vi "TLB Native Dynamic Events ver 0.13g.vi"() -> ()   [LabVIEW 2018]
uses:
  Labview Training Phase 2/Enum Controls/States for Action Engine.ctl
  TLB Type Definitions/State Type Definitions.ctl
  TLB Type Definitions/Intruction Type Definitions.ctl
  TLB Type Definitions/Encoder cluster.ctl
  TLB Type Definitions/PING CLUSTER.ctl
  <vilib>/Studica/Studica Toolkit/NavX/NavX.lvlib
  <vilib>/Studica/Studica Toolkit/Background/DIO Channel.ctl
  Underlying VI's/NavX VI/navX type def.ctl
  <vilib>/myRIO/Instrument Drivers/Utilities/Utilities.lvlib
  <vilib>/Studica/Studica Toolkit/Background/I2C Channel.ctl
  TLB Type Definitions/Vision cluster.ctl
  <vilib>/NI_Real-Time Target Support.lvlib
  TLB Type Definitions/Stepper cluster.ctl
  Experimental VI's/Archived VI's/MOTOR CONTROL NO PID Type Def.ctl
  Underlying VI's/I2C Master VI/I2C MASTER Type Def.ctl
  Underlying VI's/I2C Master VI/I2C_MASTER_WRITE_NEW Type Def.ctl
  Underlying VI's/Webcam FGV Low level ver/State control.ctl
  <vilib>/userdefined/High Color/IMAQdx.ctl
  Underlying VI's/I2C Master VI/Arduino_Interfacing.ctl
  TLB Type Definitions/Yaw Cluster.ctl
  Experimental VI's/Archived VI's/MOTOR CONTROL NO PID AE DATA ENTRY MODE Type def.ctl
  Experimental VI's/Archived VI's/MOTOR CONTROL NO PID AE DIRECTIONS type def.ctl
  Underlying VI's/Elasped Timer/Control.ctl
  TLB Type Definitions/Time cluster.ctl
  TLB Type Definitions/Y Stepper cluster.ctl
  <vilib>/Utility/RT CPU Load.ctl
panel:
  out "Time up flag":bool
  out "Recognized object + Time up?":bool
  out "Speed & distance":T1
  out "Task selection":u8
  out "Object Center Coordinates":cluster{"x":sgl, "y":sgl}
  out "Object detection cluster":T2
  in  "Object recognition mode":enum16{"Ball", "Soap", "Gel", "Pipe", "None"}(ring)
  out "NavX Readings":T3
  out "Arduino Data":T4
  out "CPU loads":T5[](array[typedef]) {"ISR (%)" format="%#.2f"; "Idle (%)" format="%#.2f"; "Background (%)" format="%#.2f"; "Normal (%)" format="%#.2f"; "Above Normal (%)" format="%#.2f"; "High (%)" format="%#.2g"; "Timed Structures (%)" format="%#.2g"; "Time Critical (%)" format="%#.2g"; "Total (%)" format="%#.2g"}
  in  "Red LED":bool
  out "Obstacle detected?":bool
  out "TASK ENABLE":bool
  out "Rising Edge":bool
  in  "Green LED":bool
  out "Obstacle detected":bool
  out "I2C Error":errorcluster
  out "State Logic":T6=enum."Startup"
  out "elements":T7[](array[typedef])
  in  "STOP TASK":bool
  in  "OK Button":bool
  in  "STOP":bool
  out "error out":errorcluster
  out "Action Queue Items":i32
  out "State Logic Queue Items":i32
  out "Action Queues items":string[](array[string])=["Hardware reset", "Software reset", ""]
  out "Action State":string
  # "System Health Status Update"
  # "TLB FRAMEWORK STATUS"
  # "Test Programme written by Calvin Loke    Dated: 28 Aug 2019\nTest Programme revised by Dr Alex See   Dated 30 Aug 2019\n\nRevision date: 19/03/2020\nProgramme version:   TLB Native Dynamic Events ver 0.13g"
  # "VISION"
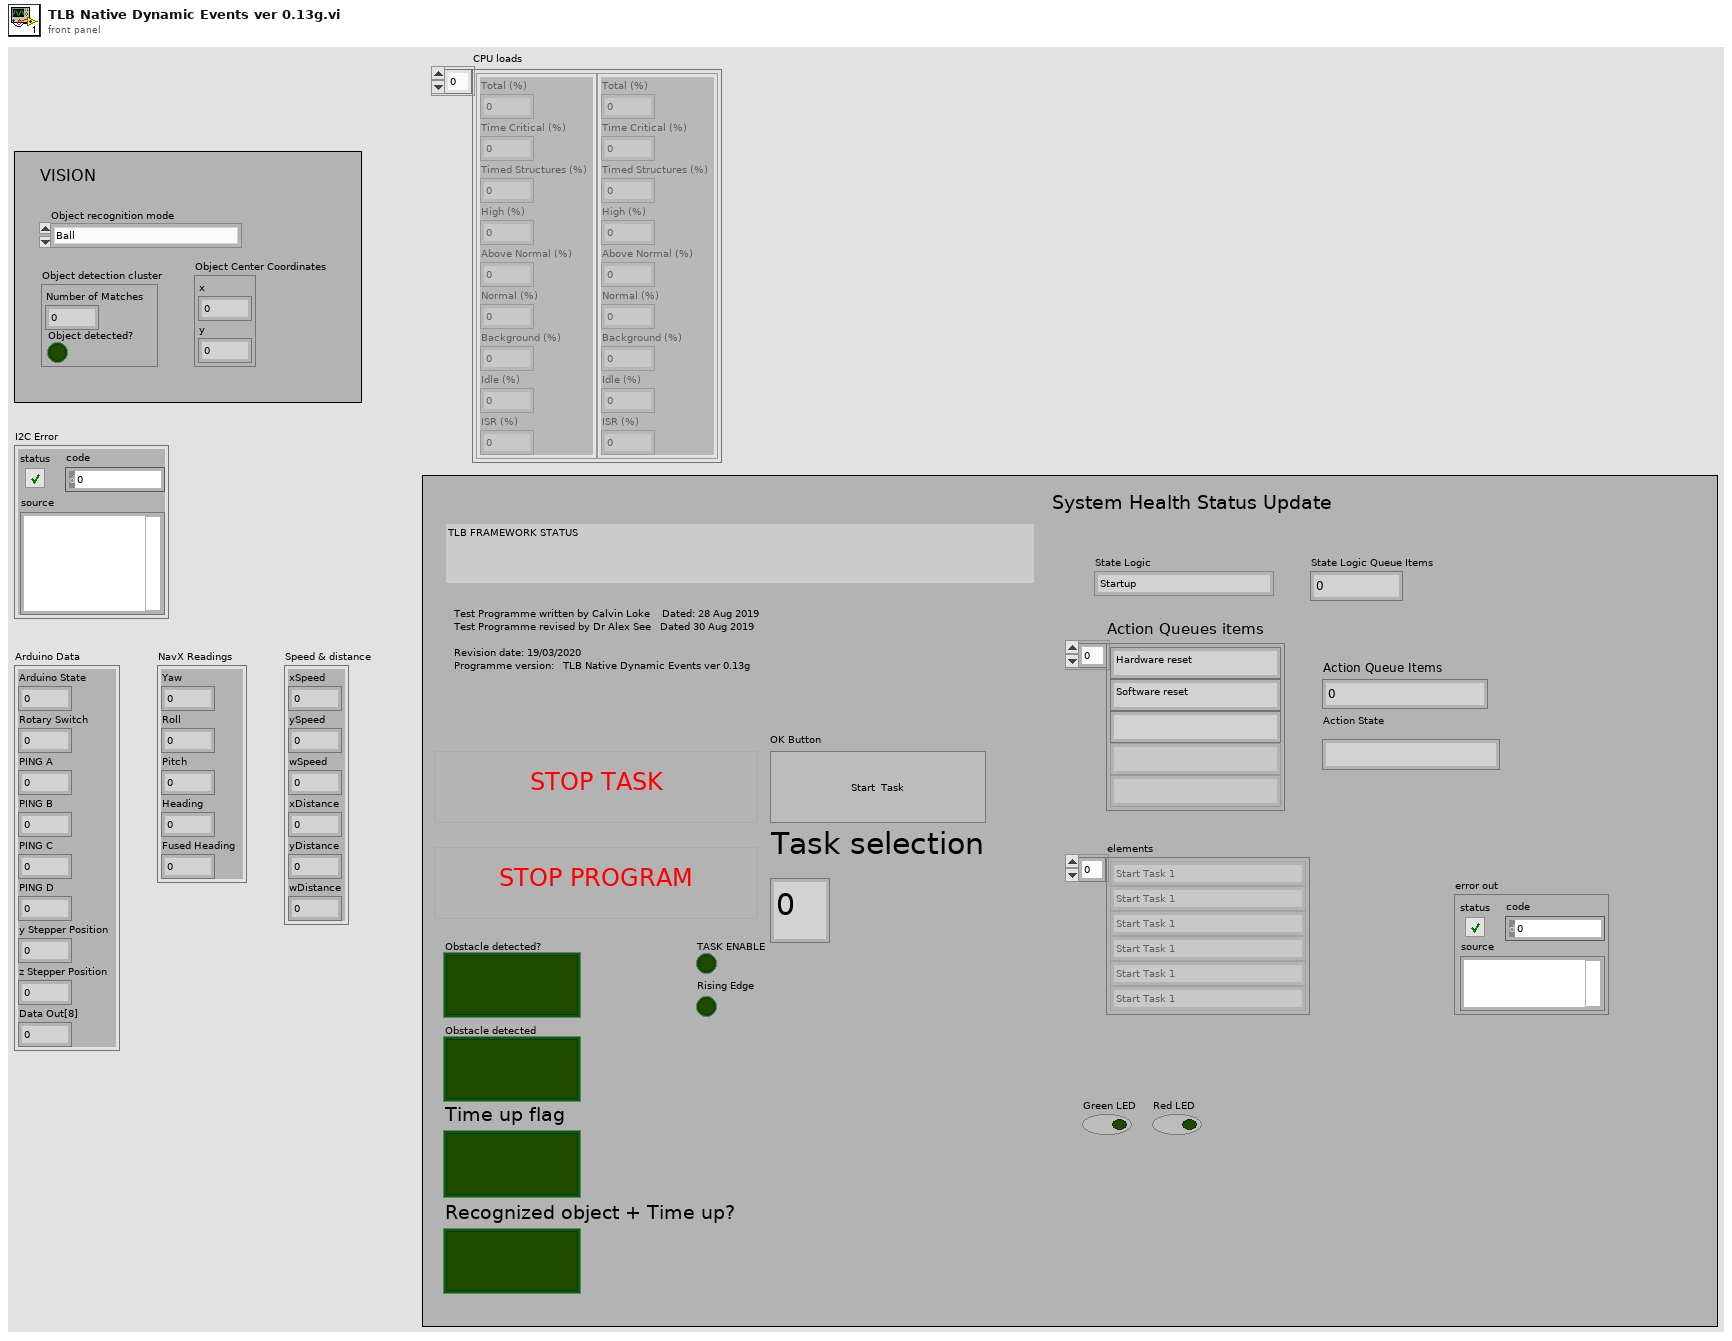
[diagram p1: front panel]
types:
  T1 = cluster{"xSpeed":dbl, "ySpeed":dbl, "wSpeed":dbl, "xDistance":dbl, "yDistance":dbl, "wDistance":dbl}
  T2 = cluster{"Number of Matches":i32, "Object detected?":bool}
  T3 = cluster{"Yaw":dbl, "Roll":dbl, "Pitch":dbl, "Heading":dbl, "Fused Heading":dbl}
  T4 = cluster{"Arduino State":u8, "Rotary Switch":u8, "PING A":u8, "PING B":u8, "PING C":u8, "PING D":u8, "y Stepper Position":u8, "z Stepper Position":u8, "Data Out[8]":u8}
  T5 = typedef "NI_Real-Time Target Support.lvlib/RT CPU Load.ctl" = cluster{"Total (%)":dbl, "Time Critical (%)":dbl, "Timed Structures (%)":dbl, "High (%)":dbl, "Above Normal (%)":dbl, "Normal (%)":dbl, "Background (%)":dbl, "Idle (%)":dbl, "ISR (%)":dbl}
  T6 = typedef "State Type Definitions.ctl" = enum16{"None", "Startup", "Move to Angle", "True Stop", "Idle", "Shutdown", "Task 1A", "Task 1B", "Task 2:Raise Arm", "Task 2:Sensor Mode", "Task 2:Reverse Mode", "Task 3", "Task 4_A", "Task 4_B", "Task 4_C", "Task 4_D", "Task 5A", "Task 5B", "Task 5C", "Task 5D", "Task 5E: POSITION ARM", "Task 5F: ARM GRAB HEIGHT", "Task 5G: CLOSE CLAW", "Task 5H: RAISE ARM", "Task 6_A", "Task 6_B", "Task 7", "Task 8A: RAISE ARM", "Task 8B: MOVE TO BOX", "Task 8C: CAM BURST", "Task 8D: PROCESS IMAGE", "Task 8E: ROBOT ADJUST", "Task 8F: CAM BURST 2", "Task 8G: PROCESS IMAGE 2", "Task 8H: ARM ADJUST", "Task 8I: ARM GRAB HEIGHT", "Task 8J: CLOSE CLAW", "Task 8K: RAISE MY SWORD", "Task 9A: Raise Arm", "Task 9B: Rotate to Angle", "Task 9C: Detect Box", "Task 9D: MOVE FORWARD", "Task 9E: MOVE LEFT", "Task 9F: SCAN IMAGE", "Task 9G: PROCESS COLOUR", "Task 9H: MOVE RIGHT", "Task 9I: SCAN IMAGE", "Task 9J: PROCESS COLOUR", "Task 9K: ROTATE 90 CW", "Task 9L: MOVE FORWARD", "Task 9M: MOVE RIGHT", "Task 9N: SCAN IMAGE", "Task 9O: PROCESS COLOUR", "Task 9P: MOVE RIGHT", "Task 9Q: SCAN IMAGE", "Task 9R: PROCESS COLOUR", "Task A1: Raise Arm", "Task A2: Rotate to Angle", "Task A3: Move Forward", "Task A4: Rotate CW 90"}
  T7 = typedef "Intruction Type Definitions.ctl" = enum16{"None", "Start Task 1", "Start Task 2", "Start Task 3", "Start Task 4", "Start Task 5", "Start Task 6", "Start Task 7", "Start Task 8 - BALL", "Start Task 8 - Gel", "Start Task 8 - Pipe", "Start Task 8 - Soap", "Start Task 9", "Start Task A", "Start Task B", "Exit"}
  T8 = typedef "Y Stepper cluster.ctl" = cluster{"yStepper desired":u8}
  T9 = typedef "Time cluster.ctl" = cluster{"Time up flag":bool, "SET TIME TO CHECK":dbl}
  T10 = typedef "Yaw Cluster.ctl" = cluster{"Yaw":dbl, "Compass":dbl}
  T11 = typedef "Stepper cluster.ctl" = cluster{"y Stepper Position":u8, "z Stepper Position":u8}
  T12 = typedef "DIO Channel.ctl" = enum16{"Not Connected", "A/DIO1", "A/DIO2", "A/DIO3", "A/DIO4", "A/DIO5", "A/DIO6", "A/DIO7", "A/DIO13", "B/DIO1", "B/DIO2", "B/DIO3", "B/DIO4", "B/DIO5", "B/DIO6", "B/DIO7", "B/DIO13", "C/DIO0", "C/DIO1", "C/DIO2", "C/DIO3", "C/DIO4", "C/DIO5", "C/DIO6", "C/DIO7"}
  T13 = typedef "Vision cluster.ctl" = cluster{"Recognized Object":bool, "Object X coordinate":dbl, "Object Y coordinate":dbl}
  T14 = typedef "PING CLUSTER.ctl" = cluster{"PING_A":u8, "PING_B":u8, "PING_C":u8, "PING_D":u8}
  T15 = typedef "Encoder cluster.ctl" = cluster{"xDistance":dbl, "yDistance":dbl, "wDistance":dbl}
  T16 = cluster{"DIO Channel":T12, "FPGA VI Reference Out":refnum<k20>}
  T17 = typedef "MOTOR CONTROL NO PID AE DATA ENTRY MODE Type def.ctl" = enum16{"Initialize", "Reset Encoders", "Write to motors", "Read from Encoders"}
  T18 = typedef "navX type def.ctl" = enum16{"Get i2C reference", "Read Values", "Zero Yaw"}
  T19 = typedef "Arduino_Interfacing.ctl" = enum16{"Initialize", "Write to Arduino", "Read From Arduino"}
  T20 = typedef "I2C Channel.ctl" = enum16{"Not Connected", "A", "B"}
  T21 = typedef "States for Action Engine.ctl" = enum16{"Initialize", "Write", "Read"}
  T22 = cluster{"I2C Ref Out":cluster{"I2C Channel":T20, "FPGA VI Reference Out":refnum<k20>}, "Connected":bool, "Slave Address (7-bit)":u8, "Registry":u8[]}
  T23 = typedef "IMAQ Image.ctl" = refnum<image>
  T24 = typedef "State Type Definitions.ctl" = enum16{"None", "Startup", "Move to Angle", "True Stop", "Idle", "Shutdown", "Task 1", "Task 2:Raise Arm", "Task 2:Sensor Mode", "Task 2:Reverse Mode", "Task 3", "Task 4_A", "Task 4_B", "Task 4_C", "Task 4_D", "Task 5A: ARM CAM HEIGHT", "Task 5B: MOVE TO BOX", "Task 5C: CAM BURST", "Task 5D: PROCESS IMAGE", "Task 5E: POSITION ARM", "Task 5F: ARM GRAB HEIGHT", "Task 5G: CLOSE CLAW", "Task 5H: RAISE ARM", "Task 6_A", "Task 6_B", "Task 7", "Task 8A: RAISE ARM", "Task 8B: MOVE TO BOX", "Task 8C: CAM BURST", "Task 8D: PROCESS IMAGE", "Task 8E: ROBOT ADJUST", "Task 8F: CAM BURST 2", "Task 8G: PROCESS IMAGE 2", "Task 8H: ARM ADJUST", "Task 8I: ARM GRAB HEIGHT", "Task 8J: CLOSE CLAW", "Task 8K: RAISE MY SWORD", "Task 9A: Raise Arm", "Task 9B: Rotate to Angle", "Task 9C: Detect Box", "Task 9D: MOVE FORWARD", "Task 9E: MOVE LEFT", "Task 9F: SCAN IMAGE", "Task 9G: PROCESS COLOUR", "Task 9H: MOVE RIGHT", "Task 9I: SCAN IMAGE", "Task 9J: PROCESS COLOUR", "Task 9K: ROTATE 90 CW", "Task 9L: MOVE FORWARD", "Task 9M: MOVE RIGHT", "Task 9N: SCAN IMAGE", "Task 9O: PROCESS COLOUR", "Task 9P: MOVE RIGHT", "Task 9Q: SCAN IMAGE", "Task 9R: PROCESS COLOUR"}
  T25 = typedef "State Type Definitions.ctl" = enum16{"None", "Startup", "Move to Angle", "True Stop", "Idle", "Shutdown", "Task 1", "Task 2", "Task 3", "Task 4_A", "Task 4_B", "Task 4_C", "Task 4_D", "Task 5_A", "Task 5 _B", "Task 5_C", "Task 5_C_Error", "Task 5_D", "Task 6_A", "Task 6_B", "Task 7", "Task 8", "Task 9", "Task A", "Task B"}
  T26 = typedef "MOTOR CONTROL NO PID AE DIRECTIONS type def.ctl" = enum16{"y-axis movement", "x-axis movement", "Rotate", "Stop"}
  T27 = typedef "Control.ctl" = enum16{"Start", "Pause", "Initialize"}
  T28 = typedef "I2C_MASTER_WRITE_NEW Type Def.ctl" = enum16{"Ultrasonic sensors", "Stepper origin", "zStepper 13.3k", "zStepper 13k", "zStepper 12k", "zStepper 11k", "zStepper 10k", "zStepper 9k", "zStepper 8k", "zStepper 7k", "zStepper 6k", "zStepper 5k", "zStepper 4k", "zStepper 3k", "zStepper 2k", "zStepper 1k", "zStepper 900", "zStepper 800", "zStepper 700", "zStepper 600", "zStepper 500", "zStepper 400", "zStepper 300", "zStepper 200", "zStepper 100", "zStepper 0", "yStepper control", "Open Claw", "Close Claw", "Soft Reset"}
  T29 = typedef "State control.ctl" = enum16{"Initialise", "Start camera", "Continuous Acquisition ", "Stop camera", "Dispose all"}
  T30 = typedef "IMAQdx.ctl" = refnum<k21>
  T31 = typedef "MOTOR CONTROL NO PID Type Def.ctl" = enum16{"Init", "Front Back", "Left Right", "Rotate", "Stop", "Latch"}
  T32 = typedef "I2C MASTER Type Def.ctl" = enum16{"Last State", "Mode 0", "Mode 1", "Mode 2", "Mode 3", "Mode 4", "Mode 5", "Mode 6", "Mode 7", "Mode 8", "Mode 9", "Mode 10"}
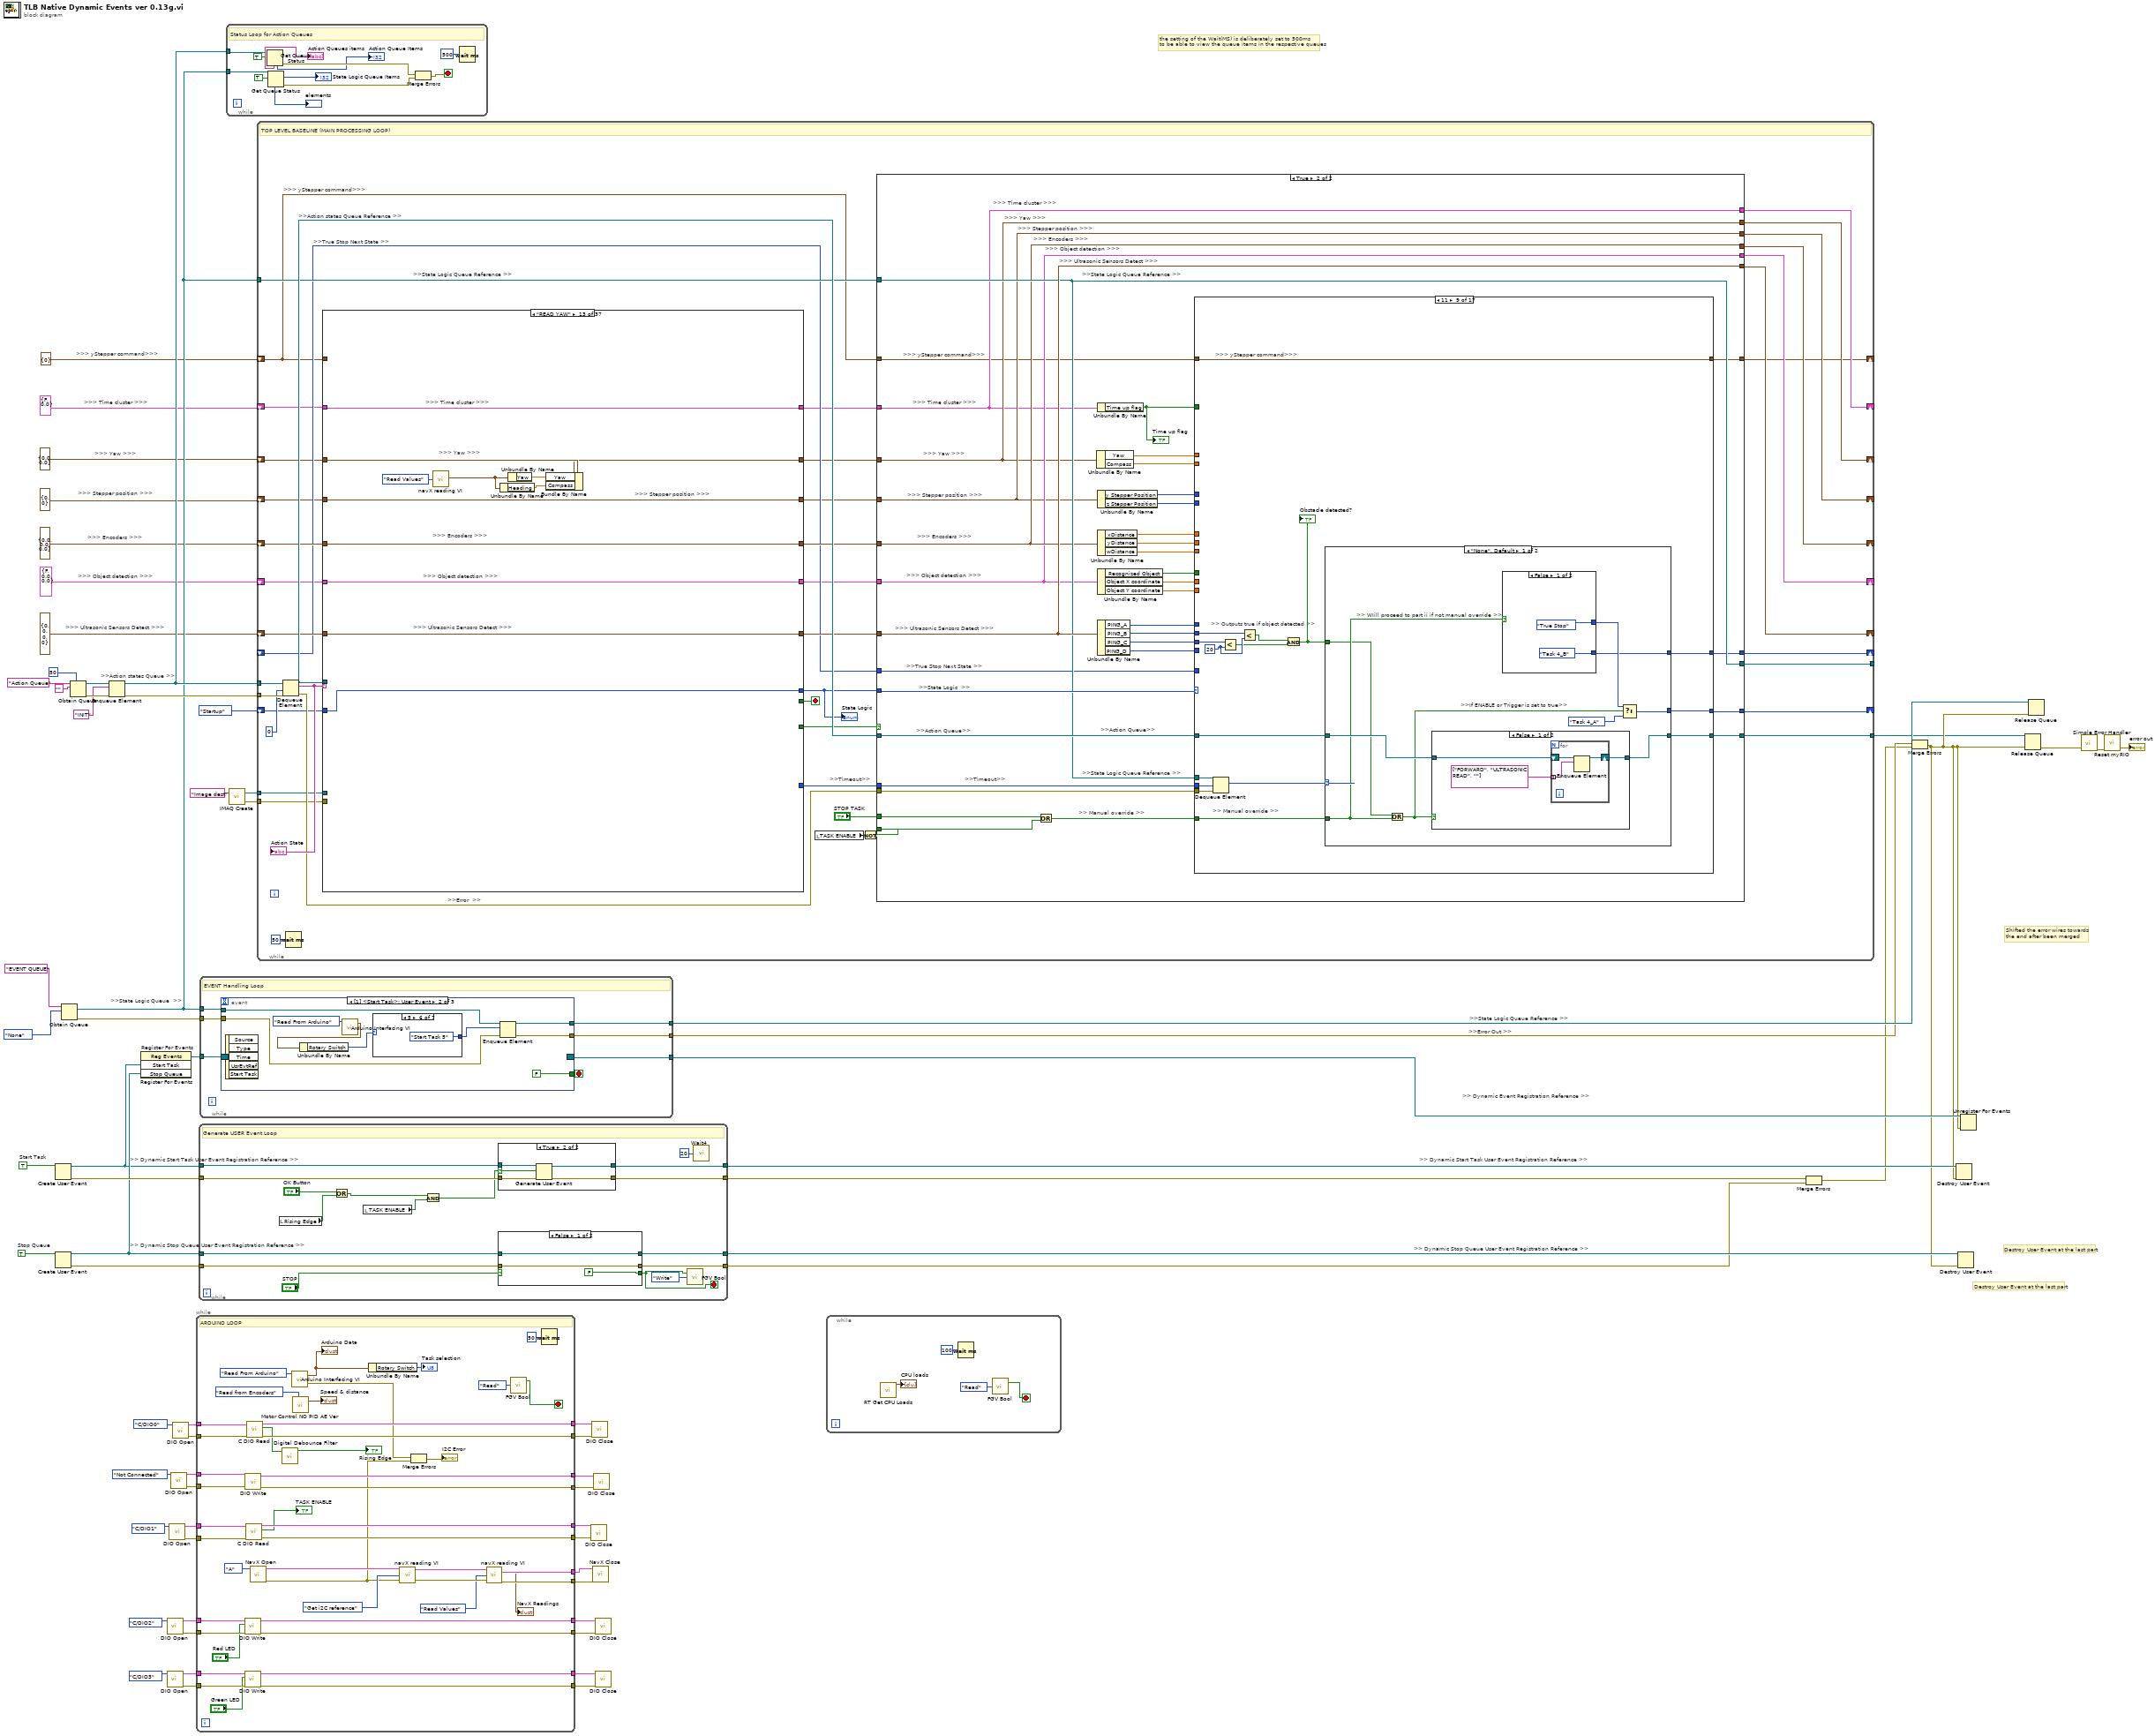
[diagram p0: block diagram]
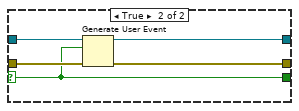
[diagram p2: hidden frame]
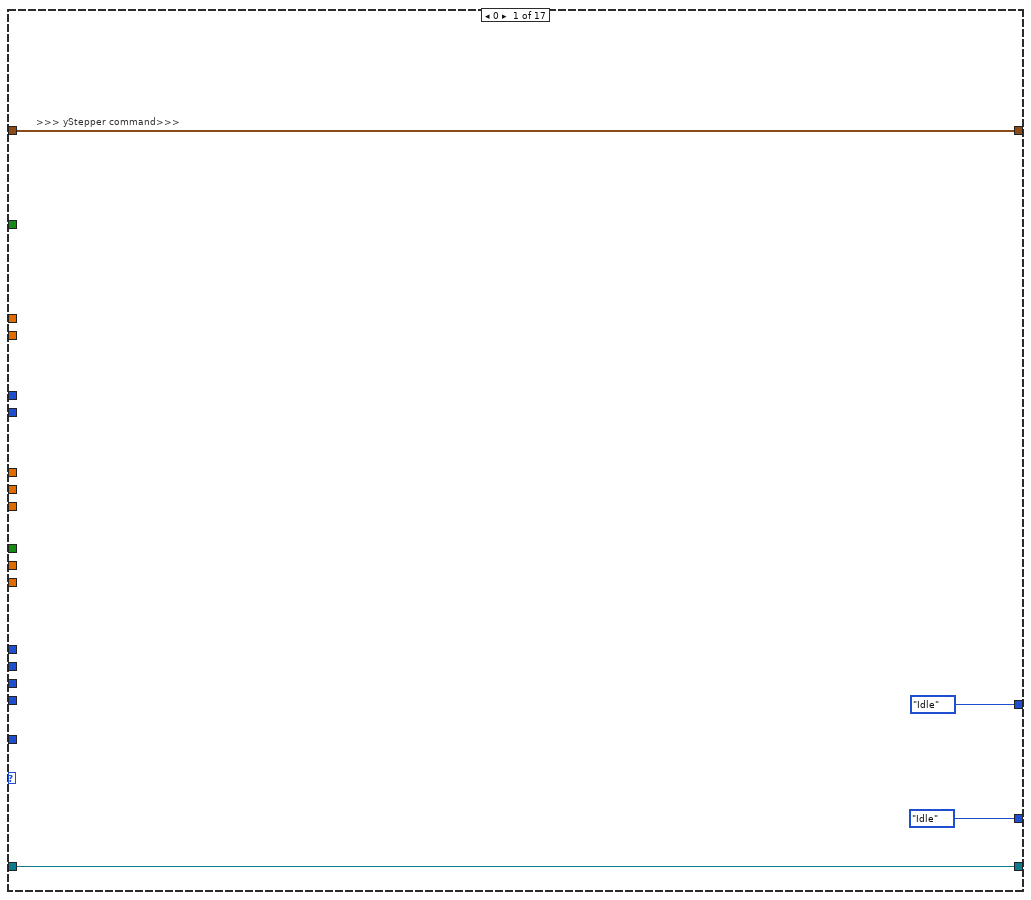
[diagram p5: hidden frame]
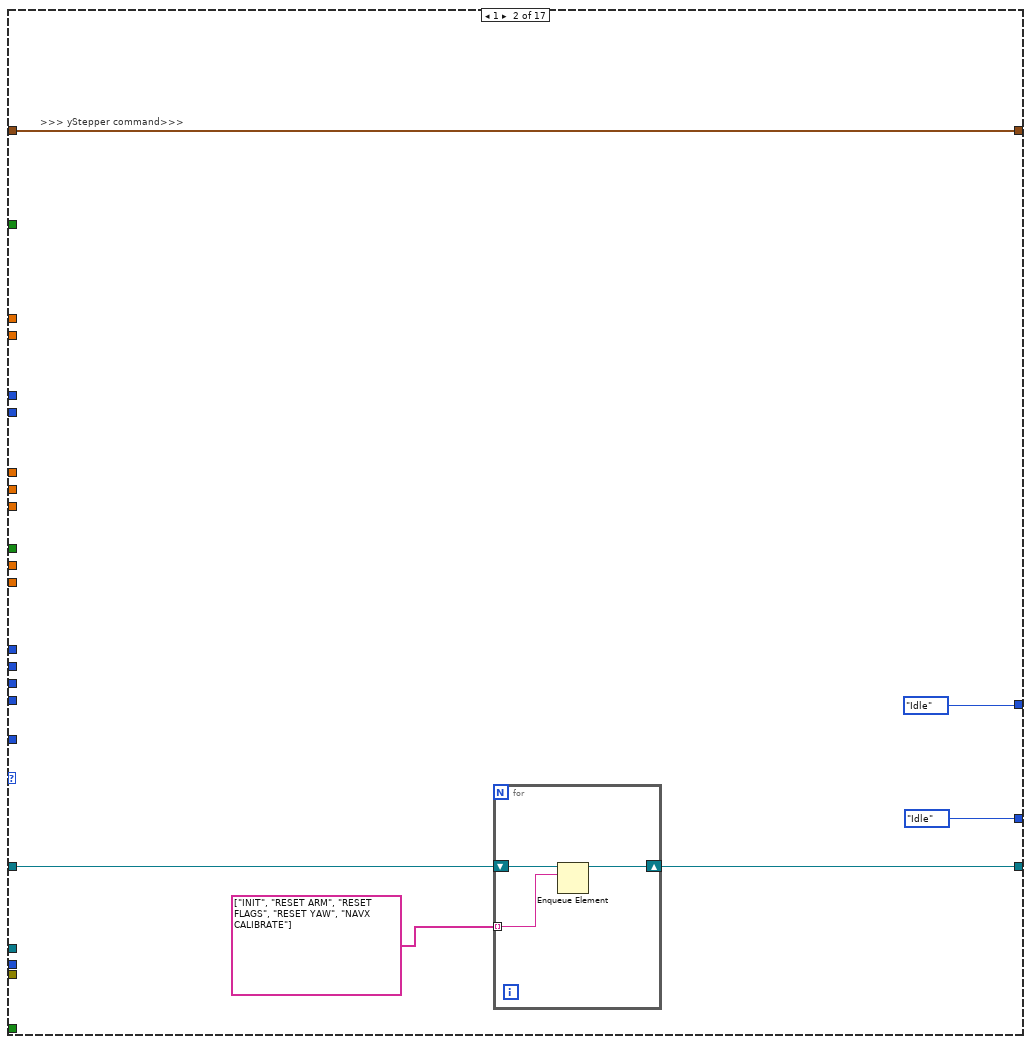
[diagram p6: hidden frame]
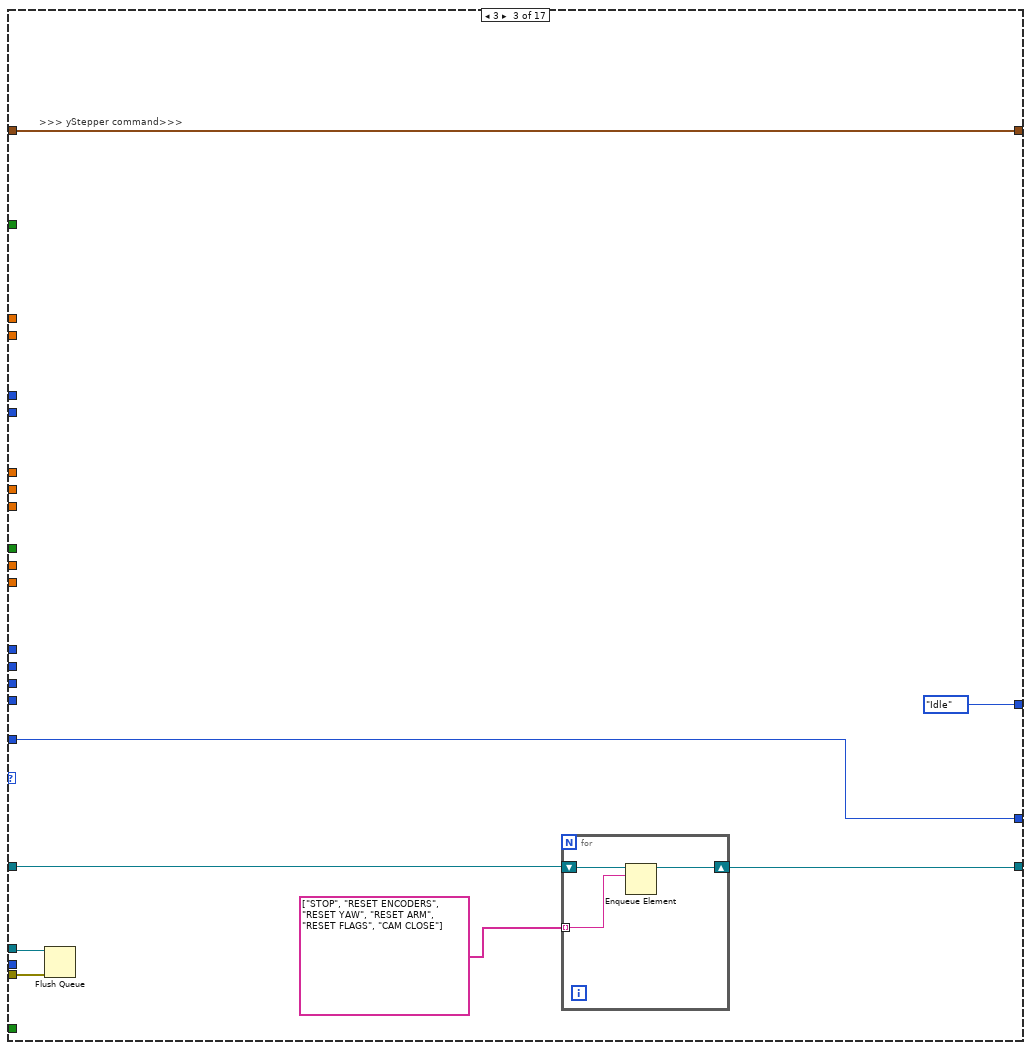
[diagram p7: hidden frame]
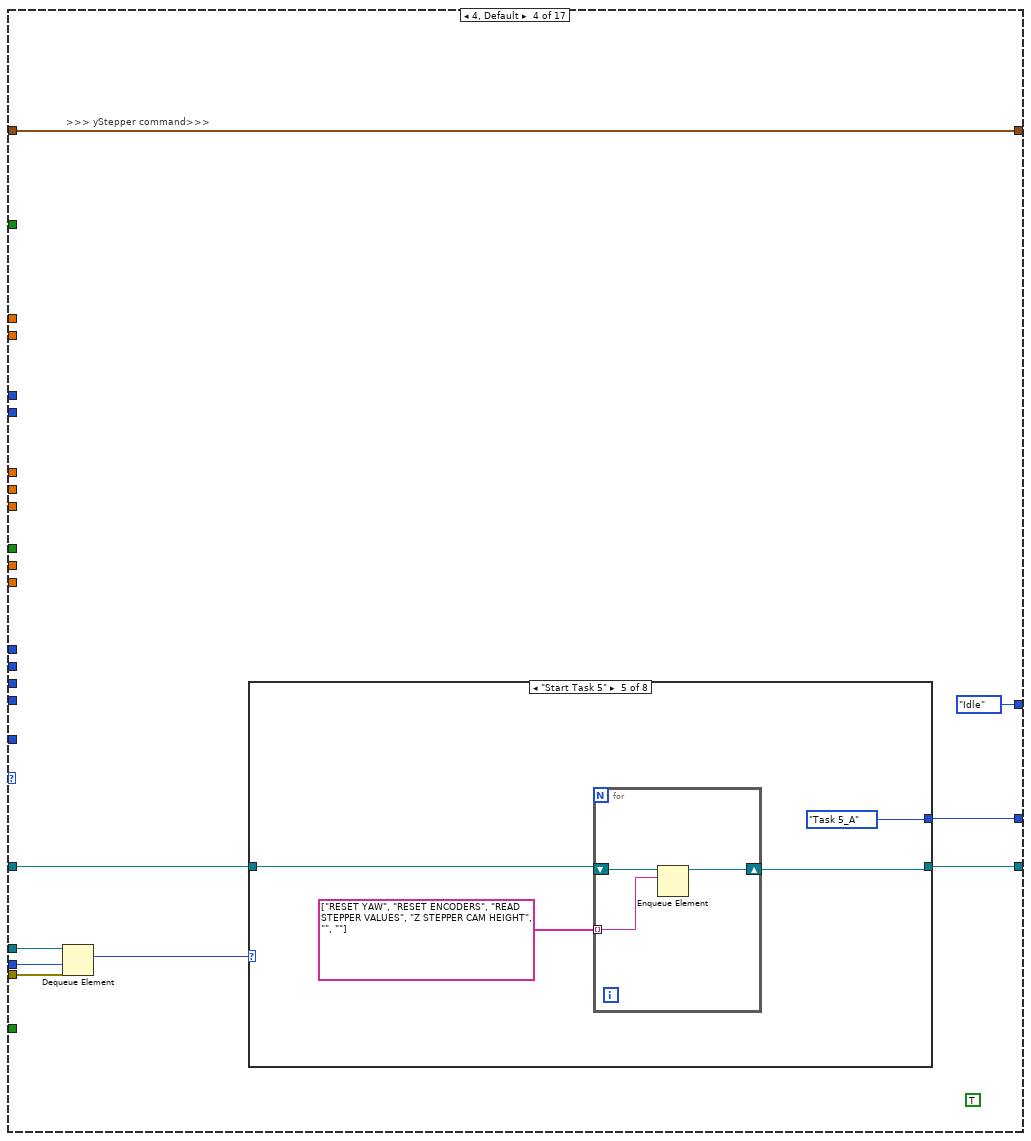
[diagram p8: hidden frame]
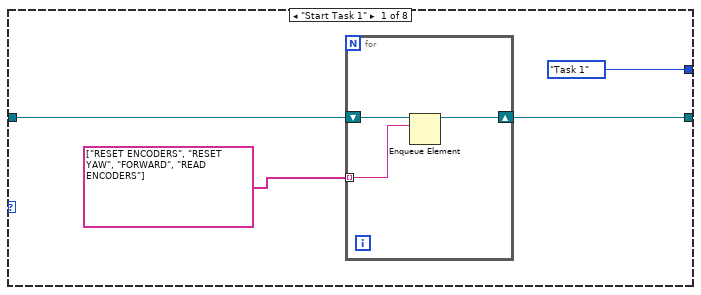
[diagram p9: hidden frame]
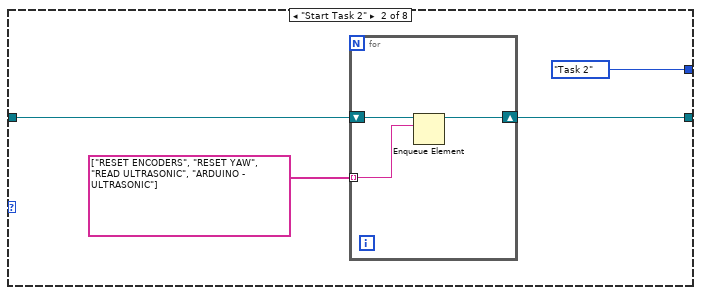
[diagram p10: hidden frame]
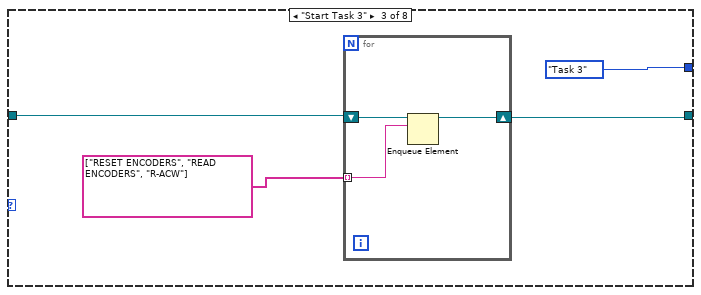
[diagram p11: hidden frame]
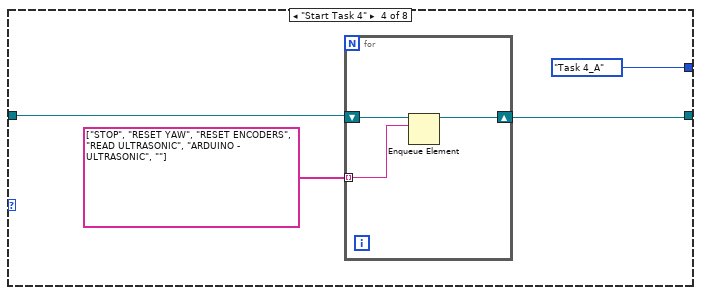
[diagram p12: hidden frame]
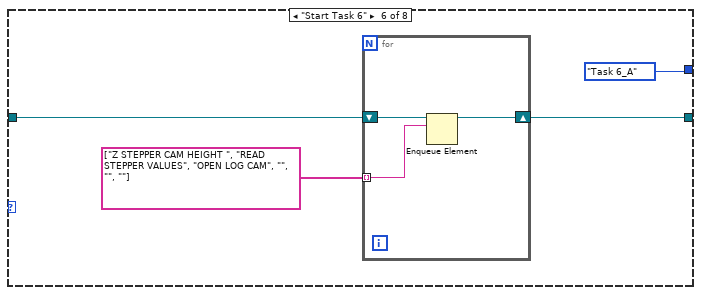
[diagram p13: hidden frame]
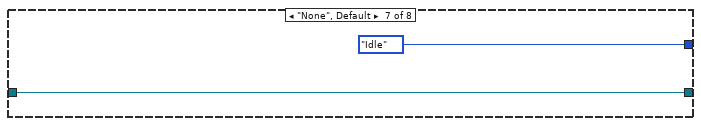
[diagram p14: hidden frame]
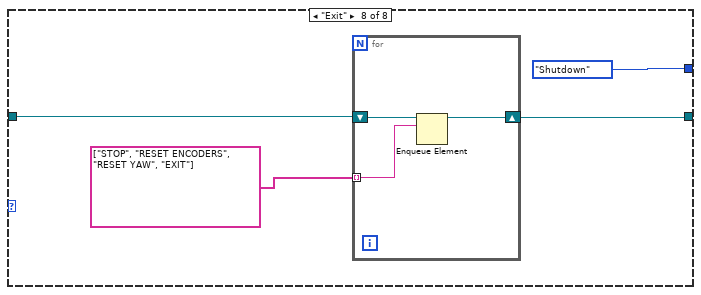
[diagram p15: hidden frame]
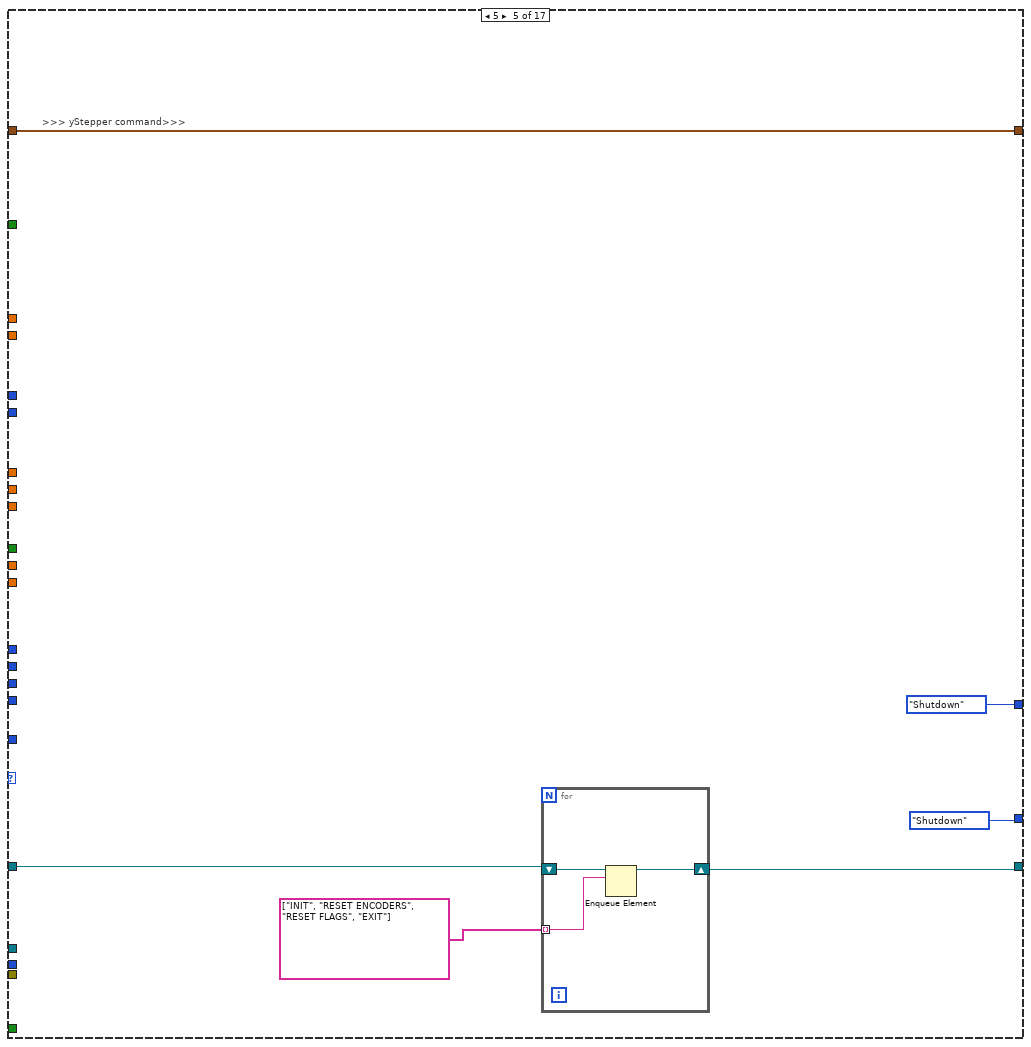
[diagram p16: hidden frame]
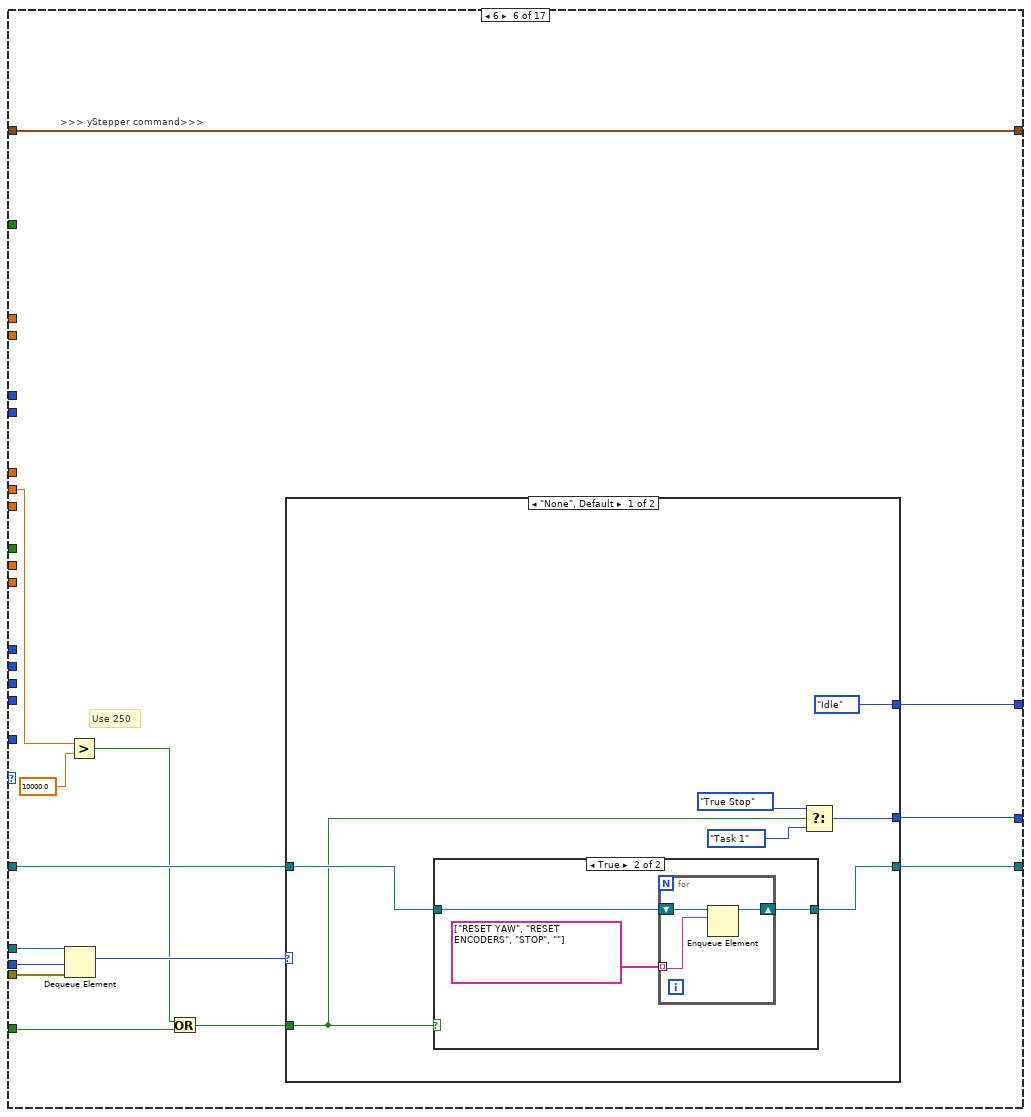
[diagram p17: hidden frame]
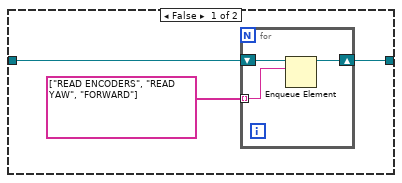
[diagram p18: hidden frame]
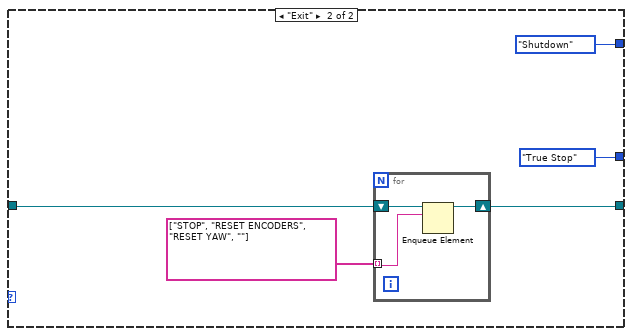
[diagram p19: hidden frame]
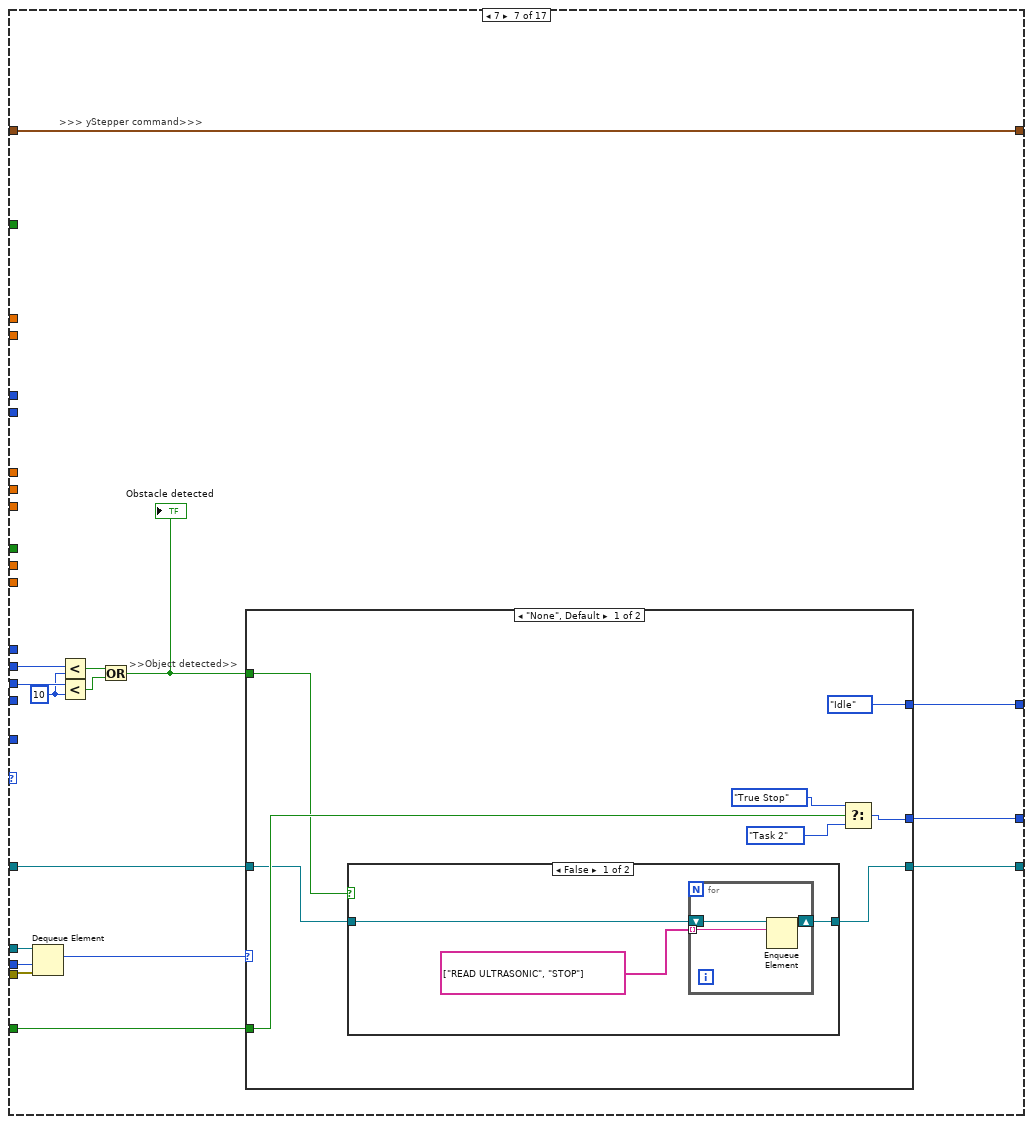
[diagram p20: hidden frame]
diagram:
  w70 = TRUE  # Stop Queue
  w69 = TRUE  # Start Task
  # ">>> yStepper command>>>"
  # ">>> Time cluster >>>"
  # ">>> Yaw >>>"
  # ">>> Stepper position >>>"
  # ">>> Encoders >>>"
  # ">>> Object detection >>>"
  # ">>> Ultrasonic Sensors Detect >>>"
  # "the setting of the Wait(MS) is deliberately set to 500ms\nto be able to view the queue items in the respective queues"
  # ">>Error Out >>"
  # ">> Dynamic Stop Queue User Event Registration Reference >>"
  # ">> Dynamic Start Task User Event Registration Reference >>"
  # ">> Dynamic Stop Queue User Event Registration Reference >>"
  # ">> Dynamic Start Task User Event Registration Reference >>"
  # ">> Dynamic Event Registration Reference >>"
  # ">>Action states Queue >>"
  # ">>State Logic Queue  >>"
  # ">>State Logic Queue Reference >>"
  # "Destroy User Event at the last part"
  # "Destroy User Event at the last part"
  # "Shifted the error wires towards\nthe end after been merged"
  n1 = Create User Event(user event datatype=w69) -> (user event=w61:refnum<user-event>, error out=w66:errorcluster)  [unwired: 1 in]
  n2 = Create User Event(user event datatype=w70) -> (user event=w62:refnum<user-event>, error out=w65:errorcluster)  [unwired: 1 in]
  n3 = Obtain Queue(name (unnamed)="EVENT QUEUE", element data type=Intruction_Type_Definitions."None" ("Enum")) -> (queue out=w47:refnum<queue>, error out=w53:errorcluster)  [unwired: 3 in, 1 out]
  n4 = Obtain Queue(max queue size (-1, unlimited)=50, name (unnamed)="Action Queue", element data type="") -> (queue out=w56:refnum<queue>, error out=w52:errorcluster)  [unwired: 2 in, 1 out]
  n5 = Enqueue Element(queue=w56, element="INIT", error in (no error)=w52) -> (queue out=w48:refnum<queue>, error out=w51:errorcluster)  [unwired: 1 in, 1 out]
  n6 = register-events "Register For Events"(w61, w62) -> (reference out=w60:refnum<event-registration>)  [unwired: 2 in, 1 out]
  n7 = call <vilib>:"DIO Open.vi"("DIO Channel"=DIO_Channel."C/DIO2") -> ("error out"=w14:errorcluster, "DIO Info Out"=w15:T16)  [unwired: 9 in]
  n8 = call <vilib>:"DIO Open.vi"("DIO Channel"=DIO_Channel."C/DIO3") -> ("error out"=w9:errorcluster, "DIO Info Out"=w10:T16)  [unwired: 9 in]
  n9 = call <vilib>:"DIO Open.vi"("DIO Channel"=DIO_Channel."C/DIO1") -> ("error out"=w25:errorcluster, "DIO Info Out"=w26:T16)  [unwired: 9 in]
  n10 = call <vilib>:"DIO Open.vi"("DIO Channel"=DIO_Channel."Not Connected") -> ("error out"=w30:errorcluster, "DIO Info Out"=w32:T16)  [unwired: 9 in]
  n11 = call <vilib>:"DIO Open.vi"("DIO Channel"=DIO_Channel."C/DIO0") -> ("error out"=w35:errorcluster, "DIO Info Out"=w38:T16)  [unwired: 9 in]
  n12 = while {
    tunnel: w38 -> [w112]
    tunnel: [w111] -> w36
    tunnel: w35 -> [w110]
    tunnel: [w109] -> w34
    tunnel: w32 -> [w105]
    tunnel: [w104] -> w31
    tunnel: w30 -> [w103]
    tunnel: [w102] -> w29
    tunnel: [w101] -> w27
    tunnel: w26 -> [w100]
    tunnel: w25 -> [w99]
    tunnel: [w98] -> w24
    tunnel: w15 -> [w92]
    tunnel: w14 -> [w91]
    tunnel: [w90] -> w13
    tunnel: [w89] -> w12
    tunnel: w10 -> [w87]
    tunnel: w9 -> [w86]
    tunnel: [w85] -> w8
    tunnel: [w84] -> w7
    tunnel: [w78] -> w4
    tunnel: [w77] -> w5
    stop <- w114 stop-if-true
    # "ARDUINO LOOP"
    n13 = call <vilib>:"DIO Write.vi"("error in (no error)"=w91, "Input"="Red LED", "DIO Info In"=w92) -> ("error out"=w89:errorcluster, "DIO Info Out"=w90:T16)  [unwired: 7 in]
    n14 = call <vilib>:"DIO Write.vi"("error in (no error)"=w86, "Input"="Green LED", "DIO Info In"=w87) -> ("error out"=w84:errorcluster, "DIO Info Out"=w85:T16)  [unwired: 7 in]
    n15 = call <vilib>:"DIO Write.vi"("error in (no error)"=w103, "DIO Info In"=w105) -> ("error out"=w102:errorcluster, "DIO Info Out"=w104:T16)  [unwired: 8 in]
    n16 = call <vilib>:"C DIO Read.vi"("error in (no error)"=w99, "DIO Info In in"=w100) -> ("error out"=w98:errorcluster, "IN"=→"TASK ENABLE":bool, "DIO Info In out"=w101:T16)  [unwired: 7 in]
    n17 = call <vilib>:"C DIO Read.vi"("error in (no error)"=w110, "DIO Info In in"=w112) -> ("error out"=w109:errorcluster, "IN"=w107:bool, "DIO Info In out"=w111:T16)  [unwired: 7 in]
    n18 = call <vilib>:"NavX Open.vi"("I2C Channel"=I2C_Channel."A") -> ("error out"=w94:errorcluster, "NavX Info"=w96:T22)  [unwired: 9 in]
    n19 = call "Digital Debounce Filter.vi"("Boolean input"=w107) -> ("Rising Edge"=→"Rising Edge":bool)  [unwired: 1 in, 2 out]
    n20 = call "Arduino Interfacing VI.vi"("AE Mode"=Arduino_Interfacing."Read From Arduino") -> ("error out"=w81:errorcluster, "Arduino Data"=w74:T4)  [unwired: 3 in]
    "Arduino Data" <- w74
    n21 = call "Motor Control NO PID AE Ver.vi"("AE Mode"=MOTOR_CONTROL_NO_PID_AE_DATA_ENTRY_MODE_Type_def."Read from Encoders") -> ("Speed & distance"=→"Speed & distance":T1)  [unwired: 4 in, 1 out]
    n22 = Unbundle By Name(w74) -> ("Rotary Switch"=→"Task selection":u8)
    n23 = call "navX reading VI.vi"("NavX Info In"=w96, "Mode"=navX_type_def."Get i2C reference", "error in (no error)"=w94) -> ("NavX Info Out"=w80:T22, "Error Out"=w79:errorcluster)  [unwired: 2 out]
    n24 = Merge Errors(w81, w94) -> (→"I2C Error":errorcluster)
    n25 = call "navX reading VI.vi"("NavX Info In"=w80, "Mode"=navX_type_def."Read Values", "error in (no error)"=w79) -> ("NavX Info Out"=w78:T22, "NavX Readings"=→"NavX Readings":T3, "Error Out"=w77:errorcluster)  [unwired: 1 out]
    n26 = call "FGV Bool.vi"("Init/Read/Write State"=States_for_Action_Engine."Read") -> ("Output node"=w114:bool)  [unwired: 2 in, 1 out]
    n27 = Wait (ms)(milliseconds to wait=u32 50) -> ()  [unwired: 1 out]
  }
  n28 = while {
    tunnel: w61 -> [w132]
    tunnel: w62 -> [w131]
    tunnel: [w130] -> w68
    tunnel: [w129] -> w67
    tunnel: w66 -> [w128]
    tunnel: [w127] -> w64
    tunnel: w65 -> [w126]
    tunnel: [w125] -> w63
    stop <- w123 stop-if-true
    # "Generate USER Event Loop"
    n29 = local read "Rising Edge"() -> (w119:bool)
    n30 = Or(x="OK Button", y=w119) -> (x .or. y?=w118:bool)
    n31 = local read "TASK ENABLE"() -> (w117:bool)
    n32 = And(x=w118, y=w117) -> (x .and. y?=w116:bool)
    n33 = case shown="True" w116 {
      selector: w116 -> [_ w143]
      tunnel: w132 -> [w142 w147]
      tunnel: [w142 w146] -> w129
      tunnel: w128 -> [w141 w145]
      tunnel: [w141 w144] -> w127
      frame False {
      }
      frame True {
        n34 = Generate User Event(user event=w147, event data cluster=w143, error in=w145) -> (user event out=w146:refnum<user-event>, error out=w144:errorcluster)  [unwired: 1 in]
      }
    }
    n35 = case shown="False" "STOP" {
      selector: "STOP" -> [_ w136]
      tunnel: w131 -> [w135 w140]
      tunnel: [w135 w139] -> w130
      tunnel: w126 -> [w134 w138]
      tunnel: [w134 w137] -> w125
      tunnel: [FALSE w136] -> w123
      frame False {
      }
      frame True {
        n36 = Generate User Event(user event=w140, event data cluster=w136, error in=w138) -> (user event out=w139:refnum<user-event>, error out=w137:errorcluster)  [unwired: 1 in]
      }
    }
    n37 = call "FGV Bool.vi"("Init/Read/Write State"=States_for_Action_Engine."Write", "Input Node"=w123) -> ()  [unwired: 1 in, 2 out]
    n38 = call "Wait4"("Count(uSec)"=u32 20) -> ()  [unwired: 1 out]
  }
  n39 = while {
    tunnel: w60 -> [w154]
    tunnel: [w153] -> w59
    tunnel: w47 -> [w151]
    tunnel: [w150] -> w58
    tunnel: w53 -> [w149]
    tunnel: [w148] -> w50
    stop <- w152 stop-if-true
    # "EVENT Handling Loop"
    n40 = event shown="[1] <Start Task>: User Event" {
      selector: w154 -> [_ _ _]
      dyn-events: [_ _ _] -> w153
      timeout: _ -> [_ _ _]
      tunnel: [FALSE FALSE w182] -> w152
      tunnel: w151 -> [w159 w168 w180]
      tunnel: [w158 w167 w181] -> w150
      tunnel: w149 -> [w157 w166 w179]
      tunnel: [w156 w165 w178] -> w148
      event Timeout {
        n41 = event-data() -> ()  [unwired: 1 in, 3 out]
        n42 = Enqueue Element(queue=w159, element=Intruction_Type_Definitions."None" ("Enum"), error in (no error)=w157) -> (queue out=w158:refnum<queue>, error out=w156:errorcluster)  [unwired: 1 in, 1 out]
      }
      event User Event {
        n43 = event-data() -> ()  [unwired: 1 in, 5 out]
        n44 = call "Arduino Interfacing VI.vi"("AE Mode"=Arduino_Interfacing."Read From Arduino") -> ("Arduino Data"=w162:T4)  [unwired: 3 in, 1 out]
        n45 = Unbundle By Name(w162) -> ("Rotary Switch"=w161:u8)
        n46 = case shown="5" w161 {
          tunnel: [Intruction_Type_Definitions."None" ("Enum") Intruction_Type_Definitions."Start Task 1" ("Enum") Intruction_Type_Definitions."Start Task 2" ("Enum") Intruction_Type_Definitions."Start Task 3" ("Enum") Intruction_Type_Definitions."Start Task 4" ("Enum") Intruction_Type_Definitions."Start Task 5" ("Enum") Intruction_Type_Definitions."Start Task 6" ("Enum")] -> w164
          frame 0, Default {
          }
          frame 1 {
          }
          frame 2 {
          }
          frame 3 {
          }
          frame 4 {
          }
          frame 5 {
          }
          frame 6 {
          }
        }
        n47 = Enqueue Element(queue=w168, element=w164, error in (no error)=w166) -> (queue out=w167:refnum<queue>, error out=w165:errorcluster)  [unwired: 1 in, 1 out]
      }
      event User Event {
        n48 = event-data() -> ("Stop Queue"=w182:bool)  [unwired: 1 in, 4 out]
        n49 = Enqueue Element At Opposite End(queue=w180, element=Intruction_Type_Definitions."Exit" ("Enum"), error in (no error)=w179) -> (queue out=w181:refnum<queue>, error out=w178:errorcluster)  [unwired: 1 in, 1 out]
      }
    }
  }
  n50 = while {
    tunnel: w48 -> [w192]
    tunnel: w47 -> [w189]
    stop <- w186 stop-if-true
    # "Status Loop for Action Queues"
    n51 = Get Queue Status(queue=w192, return elements? (F)=TRUE) -> (error out=w188:errorcluster, # elements in queue=→"Action Queue Items":i32, elements=→"Action Queues items":string[])  [unwired: 1 in, 5 out]
    n52 = Get Queue Status(queue=w189, return elements? (F)=TRUE) -> (# pending remove=→"State Logic Queue Items":i32, error out=w187:errorcluster, elements=→"elements":T7[])  [unwired: 1 in, 5 out]
    n53 = Merge Errors(w188, w187) -> (w186:errorcluster)
    n54 = Wait (ms)(milliseconds to wait=u32 500) -> ()  [unwired: 1 out]
  }
  n55 = call "IMAQ Create"("Image Name"="Image dest") -> ("New Image"=w19:T23, "error out"=w18:errorcluster)  [unwired: 4 in]
  n56 = while {
    tunnel: w47 -> [w225]
    tunnel: w48 -> [w237]
    tunnel: w51 -> [w235]
    tunnel: [w234] -> _
    tunnel: [w233] -> w41
    shift-right: [w226] -> _
    shift-left: T14 {"PING_A"=0, "PING_B"=0, "PING_C"=0, "PING_D"=0} -> [w228]
    shift-right: [w219] -> _
    shift-left: State_Type_Definitions."Startup" ("Enum") -> [w222]
    shift-right: [w215] -> _
    shift-left: T15 {"xDistance"=0.0, "yDistance"=0.0, "wDistance"=0.0} -> [w217]
    shift-right: [w212] -> _
    shift-left: _ -> [w211]
    tunnel: w19 -> [w210]
    tunnel: w18 -> [w209]
    shift-right: [w206] -> _
    shift-left: T13 {"Recognized Object"=FALSE, "Object X coordinate"=0.0, "Object Y coordinate"=0.0} -> [w208]
    shift-right: [w203] -> _
    shift-left: T11 {"y Stepper Position"=0, "z Stepper Position"=0} -> [w205]
    shift-right: [w200] -> _
    shift-left: T10 {"Yaw"=0.0, "Compass"=0.0} -> [w202]
    shift-right: [w197] -> _
    shift-left: T9 {"Time up flag"=FALSE, "SET TIME TO CHECK"=0.0} -> [w199]
    shift-right: [w195] -> _
    shift-left: T8 {"yStepper desired"=0} -> [w196]
    stop <- w224 stop-if-true
    # ">>> yStepper command>>>"
    # ">>True Stop Next State >>"
    # ">>Error  >>"
    # ">>Timeout>>"
    # ">>Action states Queue Reference >>"
    # ">>State Logic Queue Reference >>"
    # "TOP LEVEL BASELINE (MAIN PROCESSING LOOP)"
    n57 = Dequeue Element(queue=w237, timeout in ms (-1)=0, error in (no error)=w235) -> (queue out=w229:refnum<queue>, element=w236:string, error out=w230:errorcluster)  [unwired: 1 out]
    "Action State" <- w236
    n58 = Wait (ms)(milliseconds to wait=u32 50) -> ()  [unwired: 1 out]
    n59 = case shown="\"READ YAW\"" w236 {
      tunnel: [_ _ _ _ _ _ _ _ _ _ _ _ _ _ _ _ 0 w1104 _ _ _ _ _ _ _ _ _ _ _ _ _ _ _ _ _ _ _] -> w232
      tunnel: w229 -> [_ _ _ _ _ _ _ _ _ _ _ _ _ _ _ _ _ _ _ _ _ _ _ _ _ _ _ _ _ _ _ _ _ _ _ _ _]
      tunnel: w228 -> [w919 w927 w938 w949 w959 w969 w980 w991 w1001 w1007 w1021 w1034 w1045 w1053 w1077 w1086 w1096 w1105 w1113 w1121 w1150 w1160 w1167 w1175 w1187 w1199 w1224 w1235 w1241 w1250 w1259 w1268 w1276 w1291 w1296 w1307 w1317]
      tunnel: [w919 w927 w938 w949 w959 w969 w980 w991 w1001 w1007 w1021 w1035 w1045 w1053 w1078 w1086 w1096 w1105 w1113 w1121 w1149 w1160 w1167 w1175 w1187 w1199 w1224 w1235 w1241 w1250 w1259 w1268 w1276 w1291 w1296 w1307 w1317] -> w227
      tunnel: [TRUE TRUE _ _ _ _ _ _ _ _ _ _ _ _ _ _ _ _ _ _ _ _ _ _ _ _ _ _ _ _ _ _ _ _ _ _ _] -> w224
      tunnel: w222 -> [w917 w925 w937 w948 w958 w968 w979 w990 w1000 w1006 w1020 w1033 w1044 w1052 w1076 w1085 w1093 w1102 w1112 w1120 w1148 w1159 w1166 w1174 w1181 w1193 w1223 w1230 w1240 w1249 w1258 w1267 w1275 w1290 w1295 w1306 w1316]
      tunnel: [_ _ _ _ _ _ _ _ _ _ _ _ _ _ _ _ _ TRUE _ _ _ _ _ _ _ _ _ _ _ _ _ _ _ _ _ _ _] -> w221
      tunnel: [w917 w925 w937 w948 w958 w968 w979 w990 w1000 w1006 w1020 w1033 w1044 w1052 w1076 w1085 w1093 w1102 w1112 w1120 w1148 w1159 w1166 w1174 w1181 w1193 w1223 w1230 w1240 w1249 w1258 w1267 w1275 w1290 w1295 w1306 w1316] -> w220
      tunnel: w217 -> [w916 w924 w936 w947 w957 w967 w978 w989 w999 w1008 w1019 w1032 w1046 w1054 w1075 w1087 w1092 w1101 w1114 w1122 w1138 w1158 w1169 w1176 w1188 w1200 w1225 w1236 w1243 w1252 w1261 w1270 w1278 w1293 w1298 w1309 w1319]
      tunnel: [w916 w924 w936 w947 w957 w967 w978 w989 w999 w1008 w1018 w1032 w1046 w1054 w1074 w1087 w1092 w1101 w1114 w1122 w1137 w1158 w1169 w1176 w1188 w1200 w1225 w1236 w1243 w1252 w1261 w1270 w1278 w1293 w1298 w1309 w1319] -> w216
      tunnel: w210 -> [w911 _ _ _ _ _ _ _ _ _ _ _ _ _ _ _ _ _ _ _ _ _ _ _ _ _ w1218 _ _ _ _ _ _ _ _ _ _]
      tunnel: w209 -> [_ _ _ _ _ _ _ _ _ _ _ _ _ _ _ _ _ _ _ _ _ _ _ _ _ _ w1217 _ _ _ _ _ _ _ _ _ _]
      tunnel: w208 -> [w915 w923 w935 w946 w956 w966 w977 w988 w997 w1005 w1017 w1031 w1039 w1051 w1066 w1084 w1091 w1100 w1111 w1119 w1143 w1156 w1168 w1173 w1180 w1192 w1209 w1229 w1242 w1251 w1260 w1269 w1277 w1292 w1297 w1308 w1318]
      tunnel: [w915 w923 w935 w946 w956 w966 w977 w988 w997 w1005 w1017 w1031 w1039 w1051 w1065 w1084 w1091 w1100 w1111 w1119 w1142 w1156 w1168 w1173 w1180 w1192 w1213 w1229 w1242 w1251 w1260 w1269 w1277 w1292 w1297 w1308 w1318] -> w207
      tunnel: w205 -> [w914 w922 w934 w945 w955 w965 w976 w987 w996 w1004 w1016 w1030 w1047 w1050 w1071 w1083 w1090 w1099 w1110 w1118 w1133 w1155 w1165 w1172 w1179 w1191 w1212 w1228 w1239 w1248 w1257 w1266 w1279 w1289 w1299 w1310 w1320]
      tunnel: [w914 w922 w934 w945 w955 w965 w976 w987 w996 w1004 w1016 w1030 w1047 w1050 w1070 w1083 w1090 w1099 w1110 w1118 w1132 w1155 w1165 w1172 w1179 w1191 w1212 w1228 w1239 w1248 w1257 w1266 w1279 w1288 w1299 w1310 w1320] -> w204
      tunnel: w202 -> [w913 w921 w929 w940 w950 w964 w971 w982 w995 w1003 w1010 w1023 w1042 w1049 w1061 w1082 w1089 w1098 w1109 w1117 w1129 w1154 w1162 w1171 w1178 w1190 w1211 w1227 w1238 w1245 w1254 w1263 w1280 w1283 w1300 w1311 w1321]
      tunnel: [w913 w921 w929 w940 w950 w964 w971 w982 w995 w1003 w1010 w1023 w1041 w1049 w1060 w1082 w1089 w1098 w1109 w1117 w1128 w1154 w1162 w1171 w1178 w1190 w1211 w1227 w1238 w1245 w1254 w1263 w1280 w1283 w1300 w1311 w1321] -> w201
      tunnel: w199 -> [w910 w920 w930 w941 w951 w960 w972 w983 w992 w1002 w1009 w1022 w1038 w1048 w1055 w1079 w1088 w1097 w1108 w1115 w1126 w1152 w1161 w1170 w1177 w1189 w1210 w1226 w1237 w1244 w1253 w1262 w1281 w1282 w1294 w1304 w1314]
      tunnel: [w910 w920 w930 w941 w951 w960 w972 w983 w992 w1002 w1009 w1022 w1038 w1048 w1055 w1079 w1088 w1097 w1108 w1115 w1125 w1152 w1161 w1170 w1177 w1189 w1210 w1226 w1237 w1244 w1253 w1262 w1281 w1282 w1294 w1302 w1313] -> w198
      tunnel: w196 -> [_ _ _ _ _ _ _ _ _ _ _ _ _ _ _ _ _ _ _ _ _ _ _ _ _ _ _ _ _ _ _ _ w1272 _ _ _ _]
      frame "Exit" {
        # ">>State Logic  >>"
        # ">>> Time cluster >>>"
        # ">>> Yaw >>>"
        # ">>> Stepper position >>>"
        # ">>> Encoders >>>"
        # ">>> Object detection >>>"
        # ">>> Ultrasonic Sensors Detect >>>"
        n60 = call "Imaq Dispose"("All Images? (No)"=TRUE, "Image"=w911) -> ()  [unwired: 4 in, 1 out]
      }
      frame "----Movement States----" {
        # ">>State Logic  >>"
        # ">>> Time cluster >>>"
        # ">>> Yaw >>>"
        # ">>> Stepper position >>>"
        # ">>> Encoders >>>"
        # ">>> Object detection >>>"
        # ">>> Ultrasonic Sensors Detect >>>"
      }
      frame "FORWARD" {
        # ">>> Time cluster >>>"
        # ">>> Yaw >>>"
        # ">>> Stepper position >>>"
        # ">>> Encoders >>>"
        # ">>> Object detection >>>"
        # ">>> Ultrasonic Sensors Detect >>>"
        n61 = Unbundle By Name(w929) -> ("Yaw"=w928:dbl)
        n62 = call "Motor Control NO PID AE Ver.vi"("Direction"=MOTOR_CONTROL_NO_PID_AE_DIRECTIONS_type_def."y-axis movement", "AE Mode"=MOTOR_CONTROL_NO_PID_AE_DATA_ENTRY_MODE_Type_def."Write to motors", "Speed"=0.5, "Yaw"=w928) -> ()  [unwired: 1 in, 2 out]
      }
      frame "LEFT" {
        # ">>State Logic  >>"
        # ">>> Time cluster >>>"
        # ">>> Yaw >>>"
        # ">>> Stepper position >>>"
        # ">>> Encoders >>>"
        # ">>> Object detection >>>"
        # ">>> Ultrasonic Sensors Detect >>>"
        n63 = Unbundle By Name(w940) -> ("Yaw"=w939:dbl)
        n64 = call "Motor Control NO PID AE Ver.vi"("Direction"=MOTOR_CONTROL_NO_PID_AE_DIRECTIONS_type_def."x-axis movement", "AE Mode"=MOTOR_CONTROL_NO_PID_AE_DATA_ENTRY_MODE_Type_def."Write to motors", "Speed"=-0.5, "Yaw"=w939) -> ()  [unwired: 1 in, 2 out]
      }
      frame "R-ACW" {
        n65 = call "Motor Control NO PID AE Ver.vi"("Direction"=MOTOR_CONTROL_NO_PID_AE_DIRECTIONS_type_def."Rotate", "AE Mode"=MOTOR_CONTROL_NO_PID_AE_DATA_ENTRY_MODE_Type_def."Write to motors", "Speed"=0.5) -> ()  [unwired: 2 in, 2 out]
      }
      frame "R-CW" {
        (unwired) -0.2 ("Speed")
        n66 = call "Motor Control NO PID AE Ver.vi"("Direction"=MOTOR_CONTROL_NO_PID_AE_DIRECTIONS_type_def."Rotate", "AE Mode"=MOTOR_CONTROL_NO_PID_AE_DATA_ENTRY_MODE_Type_def."Write to motors", "Speed"=-0.5) -> ()  [unwired: 2 in, 2 out]
      }
      frame "RIGHT" {
        n67 = Unbundle By Name(w971) -> ("Yaw"=w970:dbl)
        n68 = call "Motor Control NO PID AE Ver.vi"("Direction"=MOTOR_CONTROL_NO_PID_AE_DIRECTIONS_type_def."x-axis movement", "AE Mode"=MOTOR_CONTROL_NO_PID_AE_DATA_ENTRY_MODE_Type_def."Write to motors", "Speed"=-0.5, "Yaw"=w970) -> ()  [unwired: 1 in, 2 out]
      }
      frame "REVERSE" {
        n69 = Unbundle By Name(w982) -> ("Yaw"=w981:dbl)
        n70 = call "Motor Control NO PID AE Ver.vi"("Direction"=MOTOR_CONTROL_NO_PID_AE_DIRECTIONS_type_def."y-axis movement", "AE Mode"=MOTOR_CONTROL_NO_PID_AE_DATA_ENTRY_MODE_Type_def."Write to motors", "Speed"=-0.5, "Yaw"=w981) -> ()  [unwired: 1 in, 2 out]
      }
      frame "STOP" {
        n71 = Wait (ms)(milliseconds to wait=u32 500) -> ()  [unwired: 1 out]
        n72 = call "Motor Control NO PID AE Ver.vi"("Direction"=MOTOR_CONTROL_NO_PID_AE_DIRECTIONS_type_def."Stop", "AE Mode"=MOTOR_CONTROL_NO_PID_AE_DATA_ENTRY_MODE_Type_def."Write to motors") -> ()  [unwired: 3 in, 2 out]
      }
      frame "----SENSOR READING---- " {
      }
      frame "READ ENCODERS" {
        # ">>> Time cluster >>>"
        # ">>> Yaw >>>"
        # ">>> Stepper position >>>"
        # ">>> Object detection >>>"
        # ">>> Current encoder distance >>>"
        # ">>> Ultrasonic Sensors Detect >>>"
        n73 = call "Motor Control NO PID AE Ver.vi"("AE Mode"=MOTOR_CONTROL_NO_PID_AE_DATA_ENTRY_MODE_Type_def."Read from Encoders") -> ("Speed & distance"=w1014:T1)  [unwired: 4 in, 1 out]
        n74 = Unbundle By Name(w1014) -> ("xDistance"=w1013:dbl, "yDistance"=w1012:dbl, "wDistance"=w1011:dbl)
        n75 = Bundle By Name(cluster=w1019, "xDistance"=w1013, "yDistance"=w1012, "wDistance"=w1011) -> (w1018:T15)
      }
      frame "READ ULTRASONIC" {
        (unwired) navX_type_def."Read Values" ("Mode")
        (unwired) MOTOR_CONTROL_NO_PID_Type_Def."Latch" ("Direction")
        # ">>> Ultrasonic Sensors Detect >>>"
        # ">>> Object detection >>>"
        # ">>> Encoders >>>"
        # ">>> Stepper position >>>"
        # ">>> Yaw >>>"
        n76 = call "Arduino Interfacing VI.vi"("AE Mode"=Arduino_Interfacing."Read From Arduino") -> ("Arduino Data"=w1028:T4)  [unwired: 3 in, 1 out]
        n77 = Unbundle By Name(w1028) -> ("PING A"=w1027:u8, "PING B"=w1026:u8, "PING C"=w1025:u8, "PING D"=w1024:u8)
        n78 = Bundle By Name(cluster=w1034, "PING_A"=w1027, "PING_B"=w1026, "PING_C"=w1025, "PING_D"=w1024) -> (w1035:T14)
      }
      frame "READ YAW" {
        # ">>> Time cluster >>>"
        # ">>> Yaw >>>"
        # ">>> Ultrasonic Sensors Detect >>>"
        # ">>> Object detection >>>"
        # ">>> Encoders >>>"
        # ">>> Stepper position >>>"
        n79 = call "navX reading VI.vi"("Mode"=navX_type_def."Read Values") -> ("NavX Readings"=w1037:T3)  [unwired: 2 in, 3 out]
        n80 = Unbundle By Name(w1037) -> ("Heading"=w1036:dbl)
        n81 = Unbundle By Name(w1037) -> ("Yaw"=w1040:dbl)
        n82 = Bundle By Name(cluster=w1042, "Yaw"=w1040, "Compass"=w1036) -> (w1041:T10)
      }
      frame "----SYSTEM MODES----" {
        (unwired) I2C_MASTER_Type_Def."Last State" ("Arduino Mode")
        # ">>> Object detection >>>"
        # ">>> Yaw >>>"
        # ">>> Ultrasonic Sensors Detect >>>"
        # ">>> Encoders >>>"
        # ">>> Stepper position >>>"
      }
      frame "INIT" {
        w1072 = u8 0
        w1073 = 0.0
        # ">>> Time cluster >>>"
        # ">>> Object detection >>>"
        # ">>> Yaw >>>"
        # ">>> Ultrasonic Sensors Detect >>>"
        # ">>> Encoders >>>"
        # ">>> Stepper position >>>"
        # ">>State Logic  >>"
        n83 = call "Arduino Interfacing VI.vi"("AE Mode"=Arduino_Interfacing."Initialize") -> ()  [unwired: 3 in, 2 out]
        n84 = call "FGV Bool.vi"("Init/Read/Write State"=States_for_Action_Engine."Initialize") -> ()  [unwired: 2 in, 2 out]
        n85 = call "Motor Control NO PID AE Ver.vi"("AE Mode"=MOTOR_CONTROL_NO_PID_AE_DATA_ENTRY_MODE_Type_def."Initialize") -> ()  [unwired: 4 in, 2 out]
        n86 = call "Elasped Timer.vi"("Action"=Control."Initialize") -> ()  [unwired: 7 in, 4 out]
        n87 = Bundle By Name(cluster=w1066, "Recognized Object"=FALSE, "Object X coordinate"=0.0, "Object Y coordinate"=0.0) -> (w1065:T13)
        n88 = Bundle By Name(cluster=w1071, "y Stepper Position"=u8 0, "z Stepper Position"=u8 0) -> (w1070:T11)
        n89 = Bundle By Name(cluster=w1075, "xDistance"=w1073, "yDistance"=w1073, "wDistance"=w1073) -> (w1074:T15)
        n90 = Bundle By Name(cluster=w1077, "PING_A"=w1072, "PING_B"=w1072, "PING_C"=w1072, "PING_D"=w1072) -> (w1078:T14)
        n91 = Bundle By Name(cluster=w1061, "Yaw"=0.0) -> (w1060:T10)
      }
      frame "ARDUINO - ULTRASONIC" {
        # ">>> Object detection >>>"
        # ">>> Yaw >>>"
        # ">>> Ultrasonic Sensors Detect >>>"
        # ">>> Encoders >>>"
        # ">>> Stepper position >>>"
        # ">>State Logic  >>"
        n92 = call "Arduino Interfacing VI.vi"("Data to Write"=I2C_MASTER_WRITE_NEW_Type_Def."Ultrasonic sensors", "AE Mode"=Arduino_Interfacing."Write to Arduino") -> ()  [unwired: 2 in, 2 out]
      }
      frame "NAVX CALIBRATE" {
        # ">>> Object detection >>>"
        # ">>> Yaw >>>"
        # ">>> Ultrasonic Sensors Detect >>>"
        # ">>> Encoders >>>"
        # ">>> Stepper position >>>"
        # ">>State Logic  >>"
        # "Adds a 15 second delay to the startup process \nfor the NavX to calibrate"
        n93 = Wait (ms)(milliseconds to wait=u32 5000) -> ()  [unwired: 1 out]
      }
      frame "NO ACTION", Default {
        (unwired) u8 0 ("y Stepper value")
        (unwired) TRUE ("Latch")
        (unwired) navX_type_def."Read Values" ("Mode")
        (unwired) MOTOR_CONTROL_NO_PID_Type_Def."Latch" ("Direction")
        # ">>> Object detection >>>"
        # ">>> Yaw >>>"
        # ">>> Ultrasonic Sensors Detect >>>"
        # ">>> Encoders >>>"
        # ">>> Stepper position >>>"
        # ">>State Logic  >>"
        n94 = case shown="4" w1102 {
          tunnel: [0 100] -> w1104
          frame 1, Default {
          }
          frame 4 {
          }
        }
      }
      frame "----RESET CASES----" {
        (unwired) I2C_MASTER_Type_Def."Last State" ("Arduino Mode")
        # ">>> Object detection >>>"
        # ">>> Yaw >>>"
        # ">>> Ultrasonic Sensors Detect >>>"
        # ">>> Encoders >>>"
        # ">>> Stepper position >>>"
        # ">>State Logic  >>"
      }
      frame "RESET ENCODERS" {
        # ">>> Object detection >>>"
        # ">>> Yaw >>>"
        # ">>> Ultrasonic Sensors Detect >>>"
        # ">>> Encoders >>>"
        # ">>> Stepper position >>>"
        # ">>State Logic  >>"
        n95 = call "Motor Control NO PID AE Ver.vi"("AE Mode"=MOTOR_CONTROL_NO_PID_AE_DATA_ENTRY_MODE_Type_def."Reset Encoders") -> ()  [unwired: 4 in, 2 out]
      }
      frame "RESET FLAGS" {
        (unwired) I2C_MASTER_Type_Def."Last State" ("Arduino Mode")
        # "Resets any software variables\nand/or non-critical states"
        n96 = Wait (ms)(milliseconds to wait=u32 20) -> ()  [unwired: 1 out]
        n97 = Bundle By Name(cluster=w1126, "Time up flag"=FALSE, "SET TIME TO CHECK"=0.0) -> (w1125:T9)
        n98 = Bundle By Name(cluster=w1143, "Recognized Object"=FALSE, "Object X coordinate"=0.0, "Object Y coordinate"=0.0) -> (w1142:T13)
        n99 = Bundle By Name(cluster=w1133, "y Stepper Position"=u8 0, "z Stepper Position"=u8 0) -> (w1132:T11)
        n100 = Bundle By Name(cluster=w1138, "xDistance"=0.0, "yDistance"=0.0, "wDistance"=0.0) -> (w1137:T15)
        n101 = Bundle By Name(cluster=w1150, "PING_A"=u8 0, "PING_B"=u8 0, "PING_C"=u8 0, "PING_D"=u8 0) -> (w1149:T14)
        n102 = Bundle By Name(cluster=w1129, "Yaw"=0.0) -> (w1128:T10)
      }
      frame "RESET YAW" {
        n103 = Wait (ms)(milliseconds to wait=u32 100) -> ()  [unwired: 1 out]
        n104 = call "navX reading VI.vi"("Mode"=navX_type_def."Zero Yaw") -> ()  [unwired: 2 in, 4 out]
      }
      frame "RESET ARM" {
        n105 = call "Arduino Interfacing VI.vi"("Data to Write"=I2C_MASTER_WRITE_NEW_Type_Def."Soft Reset", "AE Mode"=Arduino_Interfacing."Write to Arduino") -> ()  [unwired: 2 in, 2 out]
      }
      frame "--------CAM STATES-------" {
      }
      frame "OPEN LOG CAM" {
        n106 = call "Low-Level Grab.vi"("States"=State_control."Initialise", "Session In"=T30 "cam0") -> ("error out"=w1183:errorcluster, "Session Out"=w1184:T30)  [unwired: 7 in, 1 out]
        n107 = call "Low-Level Grab.vi"("error in (no error)"=w1183, "States"=State_control."Start camera", "Session In"=w1184) -> ()  [unwired: 6 in, 3 out]
      }
      frame "OPEN LIFE CAM" {
        (unwired) MOTOR_CONTROL_NO_PID_Type_Def."Latch" ("Direction")
        (unwired) navX_type_def."Read Values" ("Mode")
        n108 = call "Low-Level Grab.vi"("States"=State_control."Initialise", "Session In"=T30 "cam1") -> ("error out"=w1195:errorcluster, "Session Out"=w1196:T30)  [unwired: 7 in, 1 out]
        n109 = call "Low-Level Grab.vi"("error in (no error)"=w1195, "States"=State_control."Start camera", "Session In"=w1196) -> ()  [unwired: 6 in, 3 out]
      }
      frame "CAM ACQ" {
        # "Checks if current coordinates are zero\nif zero, take value from shift register (previous loop iteration)\nif not zero, take current value and store into shift register for subsequent loop iterations"
        # ">>> Time cluster >>>"
        # ">>> Yaw >>>"
        # ">>> Stepper position >>>"
        # ">>> Encoders >>>"
        # ">>> Object detection >>>"
        # ">>> Ultrasonic Sensors Detect >>>"
        # "Object detection"
        n110 = Unbundle By Name(w1209) -> ("Object X coordinate"=w1205:dbl, "Object Y coordinate"=w1204:dbl)
        n111 = call "Low-Level Grab.vi"("error in (no error)"=w1217, "States"=State_control."Continuous Acquisition ") -> ("error out"=w1220:errorcluster, "Image Out"=w1221:T23)  [unwired: 7 in, 1 out]
        n112 = call "Object Detection SubVI.vi"("Error In"=w1220, "Mode"="Object recognition mode", "Image Dest"=w1218, "Image in"=w1221) -> ("Object Center Coordinates"=w1216:cluster{"x":sgl, "y":sgl}, "Object detection cluster"=w1215:T2)  [unwired: 2 out]
        "Object detection cluster" <- w1215
        "Object Center Coordinates" <- w1216
        n113 = Unbundle By Name(w1215) -> ("Object detected?"=w1214:bool)
        n114 = Unbundle By Name(w1216) -> ("x"=w1202:sgl, "y"=w1201:sgl)
        n115 = Equal To 0?(x=w1202) -> (x = 0?=w1206:bool)
        n116 = Equal To 0?(x=w1201) -> (x = 0?=w1203:bool)
        n117 = Select(t=w1204, s=w1203, f=w1201) -> (s? t:f=w1207:dbl)
        n118 = Select(t=w1205, s=w1206, f=w1202) -> (s? t:f=w1208:dbl)
        n119 = Bundle By Name(cluster=w1209, "Recognized Object"=w1214, "Object X coordinate"=w1208, "Object Y coordinate"=w1207) -> (w1213:T13)
      }
      frame "CAM CLOSE" {
        n120 = call "Low-Level Grab.vi"("States"=State_control."Stop camera") -> ("error out"=w1232:errorcluster, "Session Out"=w1233:T30)  [unwired: 8 in, 1 out]
        n121 = call "Low-Level Grab.vi"("error in (no error)"=w1232, "States"=State_control."Dispose all", "Session In"=w1233) -> ()  [unwired: 6 in, 3 out]
      }
      frame "-----ARM ACTIONS-----" {
      }
      frame "CLOSE CLAW" {
        n122 = call "Arduino Interfacing VI.vi"("Data to Write"=I2C_MASTER_WRITE_NEW_Type_Def."Close Claw", "AE Mode"=Arduino_Interfacing."Write to Arduino") -> ()  [unwired: 2 in, 2 out]
      }
      frame "OPEN CLAW" {
        n123 = call "Arduino Interfacing VI.vi"("Data to Write"=I2C_MASTER_WRITE_NEW_Type_Def."Open Claw", "AE Mode"=Arduino_Interfacing."Write to Arduino") -> ()  [unwired: 2 in, 2 out]
      }
      frame "Z STEPPER CAM HEIGHT" {
        n124 = call "Arduino Interfacing VI.vi"("Data to Write"=I2C_MASTER_WRITE_NEW_Type_Def."zStepper 8k", "AE Mode"=Arduino_Interfacing."Write to Arduino") -> ()  [unwired: 2 in, 2 out]
      }
      frame "Y STEPPER CONTROL" {
        # ">>> yStepper command>>>"
        # ">>> Time cluster >>>"
        # ">>> Yaw >>>"
        # ">>> Stepper position >>>"
        # ">>> Encoders >>>"
        # ">>> Object detection >>>"
        # ">>> Ultrasonic Sensors Detect >>>"
        n125 = Unbundle By Name(w1272) -> ("yStepper desired"=w1271:u8)
        n126 = call "Arduino Interfacing VI.vi"("y Stepper value"=w1271, "Data to Write"=I2C_MASTER_WRITE_NEW_Type_Def."yStepper control", "AE Mode"=Arduino_Interfacing."Write to Arduino") -> ()  [unwired: 1 in, 2 out]
      }
      frame "READ STEPPER VALUES" {
        # ">>State Logic  >>"
        # ">>> Time cluster >>>"
        # ">>> Yaw >>>"
        # ">>> Stepper position >>>"
        # ">>> Encoders >>>"
        # ">>> Object detection >>>"
        # ">>> Ultrasonic Sensors Detect >>>"
        n127 = call "Arduino Interfacing VI.vi"("AE Mode"=Arduino_Interfacing."Read From Arduino") -> ("Arduino Data"=w1286:T4)  [unwired: 3 in, 1 out]
        n128 = Unbundle By Name(w1286) -> ("y Stepper Position"=w1285:u8, "z Stepper Position"=w1284:u8)
        n129 = Bundle By Name(cluster=w1289, "y Stepper Position"=w1285, "z Stepper Position"=w1284) -> (w1288:T11)
      }
      frame " -----TIMING-----" {
        # ">>State Logic  >>"
        # ">>> Time cluster >>>"
        # ">>> Yaw >>>"
        # ">>> Stepper position >>>"
        # ">>> Encoders >>>"
        # ">>> Object detection >>>"
        # ">>> Ultrasonic Sensors Detect >>>"
      }
      frame "SET TIMER" {
        # ">>State Logic  >>"
        # ">>> Time cluster >>>"
        # ">>> Yaw >>>"
        # ">>> Stepper position >>>"
        # ">>> Encoders >>>"
        # ">>> Object detection >>>"
        # ">>> Ultrasonic Sensors Detect >>>"
        n130 = call "Elasped Timer.vi"("Time Setting"=5.0, "Action"=Control."Initialize") -> ()  [unwired: 6 in, 4 out]
        n131 = Bundle By Name(cluster=w1304, "Time up flag"=FALSE) -> (w1302:T9)
      }
      frame "START TIMER" {
        # ">>State Logic  >>"
        # ">>> Time cluster >>>"
        # ">>> Yaw >>>"
        # ">>> Stepper position >>>"
        # ">>> Encoders >>>"
        # ">>> Object detection >>>"
        # ">>> Ultrasonic Sensors Detect >>>"
        n132 = call "Elasped Timer.vi"("Action"=Control."Start") -> ("Time Out?!"=w1312:bool)  [unwired: 7 in, 3 out]
        n133 = Bundle By Name(cluster=w1314, "Time up flag"=w1312) -> (w1313:T9)
      }
    }
    "State Logic" <- w220
    n134 = local read "TASK ENABLE"() -> (w214:bool)
    n135 = Not(x=w214) -> (.not. x?=w213:bool)
    n136 = case shown="True" w221 {
      tunnel: w225 -> [w248 w278]
      tunnel: w229 -> [w244 w280]
      tunnel: [w248 w278] -> w234
      tunnel: [w244 w281] -> w233
      tunnel: w230 -> [_ w276]
      tunnel: w232 -> [_ w277]
      tunnel: w227 -> [w247 w283]
      tunnel: [w247 w283] -> w226
      tunnel: "STOP TASK" -> [_ w266]
      tunnel: w220 -> [w246 w282]
      tunnel: [w246 w279] -> w219
      tunnel: w216 -> [w245 w272]
      tunnel: [w245 w272] -> w215
      tunnel: w213 -> [_ w267]
      tunnel: [w243 w264] -> w212
      tunnel: w211 -> [w243 w263]
      tunnel: w207 -> [w242 w260]
      tunnel: [w242 w260] -> w206
      tunnel: w204 -> [w241 w256]
      tunnel: [w241 w256] -> w203
      tunnel: w201 -> [w240 w254]
      tunnel: [w240 w254] -> w200
      tunnel: w198 -> [w239 w252]
      tunnel: [w239 w252] -> w197
      tunnel: w196 -> [w238 w251]
      tunnel: [w238 w250] -> w195
      frame False {
        # ">>> yStepper command>>>"
        # ">>> Time cluster >>>"
        # ">>> Yaw >>>"
        # ">>> Stepper position >>>"
        # ">>> Encoders >>>"
        # ">>> Object detection >>>"
        # ">>> Ultrasonic Sensors Detect >>>"
        # ">>> Time cluster >>>"
        # ">>> Yaw >>>"
        # ">>> Stepper position >>>"
        # ">>> Encoders >>>"
        # ">>> Object detection >>>"
        # ">>> Ultrasonic Sensors Detect >>>"
      }
      frame True {
        # ">>State Logic Queue Reference >>"
        # ">>Timeout>>"
        # ">>> yStepper command>>>"
        # ">>> Time cluster >>>"
        # ">>> Object detection >>>"
        # ">>> Yaw >>>"
        # ">>> Ultrasonic Sensors Detect >>>"
        # ">>> Encoders >>>"
        # ">>> Stepper position >>>"
        # ">>State Logic  >>"
        # ">>True Stop Next State >>"
        # ">>Action Queue>>"
        # ">> Manual override >>"
        # ">>> Time cluster >>>"
        # ">>> Yaw >>>"
        # ">>> Stepper position >>>"
        # ">>> Encoders >>>"
        # ">>> Object detection >>>"
        # ">>> Ultrasonic Sensors Detect >>>"
        # ">>Action Queue>>"
        # ">>State Logic Queue Reference >>"
        n137 = Or(x=w266, y=w267) -> (x .or. y?=w265:bool)
        n138 = Unbundle By Name(w254) -> ("Yaw"=w255:dbl, "Compass"=w249:dbl)
        n139 = Unbundle By Name(w252) -> ("Time up flag"=w253:bool)
        "Time up flag" <- w253
        n140 = Unbundle By Name(w256) -> ("y Stepper Position"=w258:u8, "z Stepper Position"=w257:u8)
        n141 = Unbundle By Name(w272) -> ("xDistance"=w269:dbl, "yDistance"=w270:dbl, "wDistance"=w271:dbl)
        n142 = Unbundle By Name(w260) -> ("Recognized Object"=w259:bool, "Object X coordinate"=w262:dbl, "Object Y coordinate"=w261:dbl)
        n143 = Unbundle By Name(w283) -> ("PING_A"=w275:u8, "PING_B"=w274:u8, "PING_C"=w273:u8, "PING_D"=w268:u8)
        n144 = case shown="11" w282 {
          tunnel: [w286 w290 w302 w310 w370 w383 w420 w467 w512 w570 w608 w663 w704 w746 w796 w839 w881] -> w281
          tunnel: w280 -> [w286 w293 w303 w313 w372 w384 w421 w468 w518 w563 w612 w653 w707 w752 w795 w834 w872]
          tunnel: [State_Type_Definitions."Idle" ("Enum") State_Type_Definitions."Idle" ("Enum") w298 w312 State_Type_Definitions."Shutdown" ("Enum") w385 w423 w466 w513 w569 w609 w662 w705 w753 w797 w840 w873] -> w279
          tunnel: w278 -> [_ _ w301 w316 _ w390 w433 w475 w517 w567 w613 w660 w699 w751 w793 w837 w880]
          tunnel: w277 -> [_ _ _ w315 _ w389 w432 w474 w516 w566 w605 w659 w698 w750 w792 w836 w878]
          tunnel: w276 -> [_ _ w300 w311 _ w388 w431 w473 w515 w565 w604 w661 w700 w749 w791 w835 w879]
          tunnel: w265 -> [_ _ _ _ _ w382 w422 w470 w511 w568 w610 w654 w708 w747 w794 w838 w876]
          tunnel: w275 -> [_ _ _ _ _ _ _ _ _ _ _ _ _ _ _ _ _]
          tunnel: w274 -> [_ _ _ _ _ _ w429 _ w509 w558 w615 _ _ _ _ _ _]
          tunnel: w273 -> [_ _ _ _ _ _ w428 _ w510 w559 w614 _ _ _ _ _ _]
          tunnel: w271 -> [_ _ _ _ _ _ _ w472 _ _ _ _ _ _ _ _ _]
          tunnel: w270 -> [_ _ _ _ _ w381 _ _ _ _ _ _ _ _ _ _ _]
          tunnel: w269 -> [_ _ _ _ _ _ _ _ _ w554 _ _ _ _ _ _ _]
          tunnel: w268 -> [_ _ _ _ _ _ _ _ _ _ _ _ _ _ _ _ _]
          tunnel: [State_Type_Definitions."Idle" ("Enum") State_Type_Definitions."Idle" ("Enum") State_Type_Definitions."Idle" ("Enum") State_Type_Definitions."Idle" ("Enum") State_Type_Definitions."Shutdown" ("Enum") w378 w419 w463 w504 w553 w607 w664 w706 w745 w798 w841 w874] -> w264
          tunnel: w263 -> [_ _ w298 _ _ _ _ _ _ _ _ _ _ _ _ _ _]
          tunnel: w259 -> [_ _ _ _ _ _ _ _ _ _ _ _ w703 _ _ _ w875]
          tunnel: w262 -> [_ _ _ _ _ _ _ _ _ _ _ _ _ _ _ _ _]
          tunnel: w261 -> [_ _ _ _ _ _ _ _ _ _ _ _ _ w744 w783 _ _]
          tunnel: w258 -> [_ _ _ _ _ _ _ _ _ _ _ _ _ _ w786 _ _]
          tunnel: w257 -> [_ _ _ _ _ _ _ _ _ _ _ w657 _ _ _ w833 _]
          tunnel: w255 -> [_ _ _ _ _ _ _ _ _ _ _ _ _ _ _ _ _]
          tunnel: w253 -> [_ _ _ _ _ _ _ _ _ _ _ _ w702 _ _ _ _]
          tunnel: w251 -> [w284 w288 w297 w308 w368 w377 w418 w462 w503 w551 w603 w652 w696 w740 w789 w830 w871]
          tunnel: [w284 w288 w297 w308 w368 w377 w418 w462 w503 w551 w603 w652 w696 w740 w788 w830 w871] -> w250
          tunnel: w249 -> [_ _ _ _ _ _ _ _ _ _ _ _ _ _ _ _ _]
          frame 0 {
            # ">>> yStepper command>>>"
          }
          frame 1 {
            # ">>> yStepper command>>>"
            n145 = for {
              shift-right: [w296] -> w290
              shift-left: w293 -> [w295]
              tunnel: string[] ["INIT", "RESET ARM", "RESET FLAGS", "RESET YAW", "NAVX CALIBRATE"] -> [w294] mode=indexing
              n146 = Enqueue Element(queue=w295, element=w294) -> (queue out=w296:refnum<queue>)  [unwired: 2 in, 2 out]
            }
          }
          frame 3 {
            # ">>> yStepper command>>>"
            n147 = Flush Queue(queue=w301, error in (no error)=w300) -> ()  [unwired: 3 out]
            n148 = for {
              shift-right: [w307] -> w302
              shift-left: w303 -> [w306]
              tunnel: string[] ["STOP", "RESET ENCODERS", "RESET YAW", "RESET ARM", "RESET FLAGS", "CAM CLOSE"] -> [w305] mode=indexing
              n149 = Enqueue Element(queue=w306, element=w305) -> (queue out=w307:refnum<queue>)  [unwired: 2 in, 2 out]
            }
          }
          frame 4, Default {
            (unwired) TRUE ("Green LED")
            # ">>> yStepper command>>>"
            n150 = Dequeue Element(queue=w316, timeout in ms (-1)=w315, error in (no error)=w311) -> (element=w314:T7)  [unwired: 3 out]
            n151 = case shown="\"Start Task 5\"" w314 {
              tunnel: [w318 w325 w332 w339 w346 w353 w360 w362] -> w310
              tunnel: w313 -> [w319 w326 w333 w340 w347 w354 w360 w363]
              tunnel: [State_Type_Definitions."Task 1" ("Enum") State_Type_Definitions."Task 2" ("Enum") State_Type_Definitions."Task 3" ("Enum") State_Type_Definitions."Task 4_A" ("Enum") State_Type_Definitions."Task 5_A" ("Enum") State_Type_Definitions."Task 6_A" ("Enum") State_Type_Definitions."Idle" ("Enum") State_Type_Definitions."Shutdown" ("Enum")] -> w312
              frame "Start Task 1" {
                n152 = for {
                  shift-right: [w323] -> w318
                  shift-left: w319 -> [w322]
                  tunnel: string[] ["RESET ENCODERS", "RESET YAW", "FORWARD", "READ ENCODERS"] -> [w321] mode=indexing
                  n153 = Enqueue Element(queue=w322, element=w321) -> (queue out=w323:refnum<queue>)  [unwired: 2 in, 2 out]
                }
              }
              frame "Start Task 2" {
                n154 = for {
                  shift-right: [w330] -> w325
                  shift-left: w326 -> [w329]
                  tunnel: string[] ["RESET ENCODERS", "RESET YAW", "READ ULTRASONIC", "ARDUINO - ULTRASONIC"] -> [w328] mode=indexing
                  n155 = Enqueue Element(queue=w329, element=w328) -> (queue out=w330:refnum<queue>)  [unwired: 2 in, 2 out]
                }
              }
              frame "Start Task 3" {
                n156 = for {
                  shift-right: [w337] -> w332
                  shift-left: w333 -> [w336]
                  tunnel: string[] ["RESET ENCODERS", "READ ENCODERS", "R-ACW"] -> [w335] mode=indexing
                  n157 = Enqueue Element(queue=w336, element=w335) -> (queue out=w337:refnum<queue>)  [unwired: 2 in, 2 out]
                }
              }
              frame "Start Task 4" {
                n158 = for {
                  shift-right: [w344] -> w339
                  shift-left: w340 -> [w343]
                  tunnel: string[] ["STOP", "RESET YAW", "RESET ENCODERS", "READ ULTRASONIC", "ARDUINO - ULTRASONIC", ""] -> [w342] mode=indexing
                  n159 = Enqueue Element(queue=w343, element=w342) -> (queue out=w344:refnum<queue>)  [unwired: 2 in, 2 out]
                }
              }
              frame "Start Task 5" {
                n160 = for {
                  shift-right: [w351] -> w346
                  shift-left: w347 -> [w350]
                  tunnel: string[] ["RESET YAW", "RESET ENCODERS", "READ STEPPER VALUES", "Z STEPPER CAM HEIGHT", "", ""] -> [w349] mode=indexing
                  n161 = Enqueue Element(queue=w350, element=w349) -> (queue out=w351:refnum<queue>)  [unwired: 2 in, 2 out]
                }
              }
              frame "Start Task 6" {
                n162 = for {
                  shift-right: [w358] -> w353
                  shift-left: w354 -> [w357]
                  tunnel: string[] ["Z STEPPER CAM HEIGHT ", "READ STEPPER VALUES", "OPEN LOG CAM", "", "", ""] -> [w356] mode=indexing
                  n163 = Enqueue Element(queue=w357, element=w356) -> (queue out=w358:refnum<queue>)  [unwired: 2 in, 2 out]
                }
              }
              frame "None", Default {
              }
              frame "Exit" {
                n164 = for {
                  shift-right: [w367] -> w362
                  shift-left: w363 -> [w366]
                  tunnel: string[] ["STOP", "RESET ENCODERS", "RESET YAW", "EXIT"] -> [w365] mode=indexing
                  n165 = Enqueue Element(queue=w366, element=w365) -> (queue out=w367:refnum<queue>)  [unwired: 2 in, 2 out]
                }
              }
            }
          }
          frame 5 {
            # ">>> yStepper command>>>"
            n166 = for {
              shift-right: [w376] -> w370
              shift-left: w372 -> [w375]
              tunnel: string[] ["INIT", "RESET ENCODERS", "RESET FLAGS", "EXIT"] -> [w374] mode=indexing
              n167 = Enqueue Element(queue=w375, element=w374) -> (queue out=w376:refnum<queue>)  [unwired: 2 in, 2 out]
            }
          }
          frame 6 {
            # ">>> yStepper command>>>"
            # "Use 250"
            n168 = Dequeue Element(queue=w390, timeout in ms (-1)=w389, error in (no error)=w388) -> (element=w387:T7)  [unwired: 3 out]
            n169 = Greater?(x=w381, y=10000.0) -> (0:w379:bool)
            n170 = Or(x=w379, y=w382) -> (x .or. y?=w386:bool)
            n171 = case shown="\"None\", Default" w387 {
              tunnel: w386 -> [w393 _]
              tunnel: [w397 State_Type_Definitions."True Stop" ("Enum")] -> w385
              tunnel: w384 -> [w394 w412]
              tunnel: [w392 w411] -> w383
              tunnel: [State_Type_Definitions."Idle" ("Enum") State_Type_Definitions."Shutdown" ("Enum")] -> w378
              frame "None", Default {
                n172 = case shown="True" w393 {
                  tunnel: w394 -> [w400 w406]
                  tunnel: [w399 w404] -> w392
                  frame False {
                    n173 = for {
                      shift-right: [w402] -> w399
                      shift-left: w400 -> [w403]
                      tunnel: string[] ["READ ENCODERS", "READ YAW", "FORWARD"] ("element") -> [w401] mode=indexing
                      n174 = Enqueue Element(queue=w403, element=w401) -> (queue out=w402:refnum<queue>)  [unwired: 2 in, 2 out]
                    }
                  }
                  frame True {
                    n175 = for {
                      shift-right: [w408] -> w404
                      shift-left: w406 -> [w409]
                      tunnel: string[] ["RESET YAW", "RESET ENCODERS", "STOP", ""] -> [w407] mode=indexing
                      n176 = Enqueue Element(queue=w409, element=w407) -> (queue out=w408:refnum<queue>)  [unwired: 2 in, 2 out]
                    }
                  }
                }
                n177 = Select(t=State_Type_Definitions."True Stop" ("Enum"), s=w393, f=State_Type_Definitions."Task 1" ("Enum")) -> (s? t:f=w397:u16)
              }
              frame "Exit" {
                n178 = for {
                  shift-right: [w416] -> w411
                  shift-left: w412 -> [w417]
                  tunnel: string[] ["STOP", "RESET ENCODERS", "RESET YAW", ""] -> [w415] mode=indexing
                  n179 = Enqueue Element(queue=w417, element=w415) -> (queue out=w416:refnum<queue>)  [unwired: 2 in, 2 out]
                }
              }
            }
          }
          frame 7 {
            w427 = u8 10 ("y")
            # ">>> yStepper command>>>"
            # ">>Object detected>>"
            n180 = Dequeue Element(queue=w433, timeout in ms (-1)=w432, error in (no error)=w431) -> (element=w430:T7)  [unwired: 3 out]
            n181 = Less?(x=w429, y=w427) -> (x < y?=w426:bool)
            n182 = Less?(x=w428, y=w427) -> (x < y?=w425:bool)
            n183 = Or(x=w426, y=w425) -> (x .or. y?=w424:bool)
            "Obstacle detected" <- w424
            n184 = case shown="\"None\", Default" w430 {
              tunnel: w424 -> [w437 _]
              tunnel: [w439 State_Type_Definitions."True Stop" ("Enum")] -> w423
              tunnel: w422 -> [w438 _]
              tunnel: w421 -> [w436 w456]
              tunnel: [w435 w457] -> w420
              tunnel: [State_Type_Definitions."Idle" ("Enum") State_Type_Definitions."Shutdown" ("Enum")] -> w419
              frame "None", Default {
                n185 = case shown="False" w437 {
                  tunnel: w436 -> [w443 w450]
                  tunnel: [w444 w449] -> w435
                  frame False {
                    n186 = for {
                      tunnel: string[] ["READ ULTRASONIC", "STOP"] ("element") -> [w445] mode=indexing
                      shift-right: [w447] -> w444
                      shift-left: w443 -> [w446]
                      n187 = Enqueue Element(queue=w446, element=w445) -> (queue out=w447:refnum<queue>)  [unwired: 2 in, 2 out]
                    }
                  }
                  frame True {
                    n188 = for {
                      shift-right: [w452] -> w449
                      shift-left: w450 -> [w453]
                      tunnel: string[] ["REVERSE", "READ ULTRASONIC"] -> [w451] mode=indexing
                      n189 = Enqueue Element(queue=w453, element=w451) -> (queue out=w452:refnum<queue>)  [unwired: 2 in, 2 out]
                    }
                  }
                }
                n190 = Select(t=State_Type_Definitions."True Stop" ("Enum"), s=w438, f=State_Type_Definitions."Task 2" ("Enum")) -> (s? t:f=w439:u16)
              }
              frame "Exit" {
                n191 = for {
                  shift-right: [w460] -> w457
                  shift-left: w456 -> [w461]
                  tunnel: string[] ["STOP", "RESET ENCODERS", "RESET YAW", "ARDUINO MODE 0"] -> [w459] mode=indexing
                  n192 = Enqueue Element(queue=w461, element=w459) -> (queue out=w460:refnum<queue>)  [unwired: 2 in, 2 out]
                }
              }
            }
          }
          frame 10 {
            # ">>> yStepper command>>>"
            n193 = Dequeue Element(queue=w475, timeout in ms (-1)=w474, error in (no error)=w473) -> (element=w464:T7)  [unwired: 3 out]
            n194 = Greater?(x=w472, y=150.0) -> (0:w469:bool)
            n195 = Or(x=w469, y=w470) -> (x .or. y?=w465:bool)
            n196 = case shown="\"Exit\"" w464 {
              tunnel: w465 -> [w478 _]
              tunnel: [w482 State_Type_Definitions."True Stop" ("Enum")] -> w466
              tunnel: w468 -> [w479 w498]
              tunnel: [w477 w497] -> w467
              tunnel: [State_Type_Definitions."Idle" ("Enum") State_Type_Definitions."Shutdown" ("Enum")] -> w463
              frame "None", Default {
                n197 = case shown="False" w478 {
                  tunnel: w479 -> [w485 w491]
                  tunnel: [w484 w489] -> w477
                  frame False {
                    n198 = for {
                      shift-right: [w487] -> w484
                      shift-left: w485 -> [w488]
                      tunnel: string[] ["READ ENCODERS", "R-ACW"] ("element") -> [w486] mode=indexing
                      n199 = Enqueue Element(queue=w488, element=w486) -> (queue out=w487:refnum<queue>)  [unwired: 2 in, 2 out]
                    }
                  }
                  frame True {
                    n200 = for {
                      shift-right: [w493] -> w489
                      shift-left: w491 -> [w494]
                      tunnel: string[] ["RESET YAW", "RESET ENCODERS", "STOP", "ARDUINO MODE 0"] -> [w492] mode=indexing
                      n201 = Enqueue Element(queue=w494, element=w492) -> (queue out=w493:refnum<queue>)  [unwired: 2 in, 2 out]
                    }
                  }
                }
                n202 = Select(t=State_Type_Definitions."True Stop" ("Enum"), s=w478, f=State_Type_Definitions."Task 3" ("Enum")) -> (s? t:f=w482:T6)
              }
              frame "Exit" {
                n203 = for {
                  shift-right: [w501] -> w497
                  shift-left: w498 -> [w502]
                  tunnel: string[] ["STOP", "RESET ENCODERS", "RESET YAW", ""] -> [w500] mode=indexing
                  n204 = Enqueue Element(queue=w502, element=w500) -> (queue out=w501:refnum<queue>)  [unwired: 2 in, 2 out]
                }
              }
            }
          }
          frame 11 {
            w508 = u8 20
            # ">>> yStepper command>>>"
            # ">> Outputs true if object detected >>"
            # ">> Manual override >>"
            n205 = Dequeue Element(queue=w517, timeout in ms (-1)=w516, error in (no error)=w515) -> (element=w514:T7)  [unwired: 3 out]
            n206 = Less?(x=w510, y=w508) -> (x < y?=w506:bool)
            n207 = Less?(x=w509, y=w508) -> (x < y?=w507:bool)
            n208 = And(x=w507, y=w506) -> (x .and. y?=w505:bool)
            "Obstacle detected?" <- w505
            n209 = case shown="\"None\", Default" w514 {
              tunnel: [w527 State_Type_Definitions."True Stop" ("Enum")] -> w513
              tunnel: [w525 w546] -> w512
              tunnel: w518 -> [w524 _]
              tunnel: w511 -> [w522 _]
              tunnel: w505 -> [w520 _]
              tunnel: [w519 State_Type_Definitions."Shutdown" ("Enum")] -> w504
              frame "None", Default {
                # ">> WIill proceed to part ii if not manual override >>"
                # ">>If ENABLE or Trigger is set to true>>"
                n210 = Or(x=w520, y=w522) -> (x .or. y?=w521:bool)
                n211 = case shown="False" w521 {
                  tunnel: [w534 w539] -> w525
                  tunnel: w524 -> [w532 w538]
                  frame False {
                    n212 = for {
                      shift-right: [w536] -> w534
                      shift-left: w532 -> [w537]
                      tunnel: string[] ["FORWARD", "ULTRASONIC READ", ""] ("element") -> [w535] mode=indexing
                      n213 = Enqueue Element(queue=w537, element=w535) -> (queue out=w536:refnum<queue>)  [unwired: 2 in, 2 out]
                    }
                  }
                  frame True {
                    n214 = for {
                      shift-right: [w542] -> w539
                      shift-left: w538 -> [w543]
                      tunnel: string[] ["STOP", "RESET ENCODERS", "RESET YAW", "ARDUINO MODE 0"] -> [w541] mode=indexing
                      n215 = Enqueue Element(queue=w543, element=w541) -> (queue out=w542:refnum<queue>)  [unwired: 2 in, 2 out]
                    }
                  }
                }
                n216 = case shown="False" w522 {
                  tunnel: [State_Type_Definitions."True Stop" ("Enum") State_Type_Definitions."True Stop" ("Enum")] -> w523
                  tunnel: [State_Type_Definitions."Task 4_B" ("Enum") State_Type_Definitions."Idle" ("Enum")] -> w519
                  frame False {
                  }
                  frame True {
                  }
                }
                n217 = Select(t=w523, s=w521, f=State_Type_Definitions."Task 4_A" ("Enum")) -> (s? t:f=w527:T6)
              }
              frame "Exit" {
                n218 = for {
                  shift-right: [w549] -> w546
                  shift-left: _ -> [w550]
                  tunnel: string[] ["STOP", "RESET ENCODERS", "RESET YAW", ""] -> [w548] mode=indexing
                  n219 = Enqueue Element(queue=w550, element=w548) -> (queue out=w549:refnum<queue>)  [unwired: 2 in, 2 out]
                }
              }
            }
          }
          frame 12 {
            w562 = 20
            # ">>> yStepper command>>>"
            # ">> Outputs true if 150 mm has been moved >>"
            # ">> Outputs true if sensor not obstructed>>"
            # ">> Manual override >>"
            n220 = Dequeue Element(queue=w567, timeout in ms (-1)=w566, error in (no error)=w565) -> (element=w564:T7)  [unwired: 3 out]
            n221 = Greater?(x=w559, y=w562) -> (0:w560:bool)
            n222 = Greater?(x=w558, y=w562) -> (0:w561:bool)
            n223 = Greater Or Equal?(x=w554, y=80.0) -> (x >= y?=w556:bool)
            n224 = And(x=w561, y=w560) -> (x .and. y?=w555:bool)
            n225 = And(x=w556, y=w555) -> (x .and. y?=w552:bool)
            n226 = case shown="\"None\", Default" w564 {
              tunnel: [w579 State_Type_Definitions."True Stop" ("Enum")] -> w569
              tunnel: [w577 w598] -> w570
              tunnel: w563 -> [w576 _]
              tunnel: w568 -> [w574 _]
              tunnel: w552 -> [w572 _]
              tunnel: [w571 State_Type_Definitions."Shutdown" ("Enum")] -> w553
              frame "None", Default {
                # ">> WIill proceed to part ii if not manual override >>"
                # ">>If ENABLE or Trigger is set to true>>"
                n227 = Or(x=w572, y=w574) -> (x .or. y?=w573:bool)
                n228 = case shown="False" w573 {
                  tunnel: [w586 w591] -> w577
                  tunnel: w576 -> [w584 w590]
                  frame False {
                    n229 = for {
                      shift-right: [w588] -> w586
                      shift-left: w584 -> [w589]
                      tunnel: string[] ["RIGHT", "ULTRASONIC READ", "READ ENCODERS"] ("element") -> [w587] mode=indexing
                      n230 = Enqueue Element(queue=w589, element=w587) -> (queue out=w588:refnum<queue>)  [unwired: 2 in, 2 out]
                    }
                  }
                  frame True {
                    n231 = for {
                      shift-right: [w594] -> w591
                      shift-left: w590 -> [w595]
                      tunnel: string[] ["STOP", "RESET ENCODERS", "RESET YAW", "ARDUINO MODE 0"] -> [w593] mode=indexing
                      n232 = Enqueue Element(queue=w595, element=w593) -> (queue out=w594:refnum<queue>)  [unwired: 2 in, 2 out]
                    }
                  }
                }
                n233 = case shown="True" w574 {
                  tunnel: [State_Type_Definitions."True Stop" ("Enum") State_Type_Definitions."True Stop" ("Enum")] -> w575
                  tunnel: [State_Type_Definitions."Task 4_C" ("Enum") State_Type_Definitions."Idle" ("Enum")] -> w571
                  frame False {
                  }
                  frame True {
                  }
                }
                n234 = Select(t=w575, s=w573, f=State_Type_Definitions."Task 4_B" ("Enum")) -> (s? t:f=w579:T6)
              }
              frame "Exit" {
                n235 = for {
                  shift-right: [w601] -> w598
                  shift-left: _ -> [w602]
                  tunnel: string[] ["STOP", "RESET ENCODERS", "RESET YAW", ""] -> [w600] mode=indexing
                  n236 = Enqueue Element(queue=w602, element=w600) -> (queue out=w601:refnum<queue>)  [unwired: 2 in, 2 out]
                }
              }
            }
          }
          frame 13 {
            w618 = u8 20
            # ">>> yStepper command>>>"
            # ">> Outputs true if object detected >>"
            # ">> Manual override >>"
            n237 = Dequeue Element(queue=w613, timeout in ms (-1)=w605, error in (no error)=w604) -> (element=w606:T7)  [unwired: 3 out]
            n238 = Less?(x=w614, y=w618) -> (x < y?=w616:bool)
            n239 = Less?(x=w615, y=w618) -> (x < y?=w617:bool)
            n240 = And(x=w617, y=w616) -> (x .and. y?=w611:bool)
            n241 = case shown="\"None\", Default" w606 {
              tunnel: [w627 State_Type_Definitions."True Stop" ("Enum")] -> w609
              tunnel: [w625 w647] -> w608
              tunnel: w612 -> [w624 w644]
              tunnel: w610 -> [w622 _]
              tunnel: w611 -> [w620 _]
              tunnel: [w619 State_Type_Definitions."Shutdown" ("Enum")] -> w607
              frame "None", Default {
                # ">> WIill proceed to part ii if not manual override >>"
                # ">>If ENABLE or Trigger is set to true>>"
                n242 = Or(x=w620, y=w622) -> (x .or. y?=w621:bool)
                n243 = case shown="False" w621 {
                  tunnel: [w634 w639] -> w625
                  tunnel: w624 -> [w632 w638]
                  frame False {
                    n244 = for {
                      shift-right: [w636] -> w634
                      shift-left: w632 -> [w637]
                      tunnel: string[] ["FORWARD", "ULTRASONIC READ", ""] ("element") -> [w635] mode=indexing
                      n245 = Enqueue Element(queue=w637, element=w635) -> (queue out=w636:refnum<queue>)  [unwired: 2 in, 2 out]
                    }
                  }
                  frame True {
                    n246 = for {
                      shift-right: [w642] -> w639
                      shift-left: w638 -> [w643]
                      tunnel: string[] ["STOP", "RESET ENCODERS", "RESET YAW", "ARDUINO MODE 0"] -> [w641] mode=indexing
                      n247 = Enqueue Element(queue=w643, element=w641) -> (queue out=w642:refnum<queue>)  [unwired: 2 in, 2 out]
                    }
                  }
                }
                n248 = case shown="True" w622 {
                  tunnel: [State_Type_Definitions."True Stop" ("Enum") State_Type_Definitions."True Stop" ("Enum")] -> w623
                  tunnel: [State_Type_Definitions."Idle" ("Enum") State_Type_Definitions."Idle" ("Enum")] -> w619
                  frame False {
                  }
                  frame True {
                  }
                }
                n249 = Select(t=w623, s=w621, f=State_Type_Definitions."Task 4_C" ("Enum")) -> (s? t:f=w627:T6)
              }
              frame "Exit" {
                n250 = for {
                  shift-right: [w650] -> w647
                  shift-left: w644 -> [w651]
                  tunnel: string[] ["STOP", "RESET ENCODERS", "RESET YAW", ""] -> [w649] mode=indexing
                  n251 = Enqueue Element(queue=w651, element=w649) -> (queue out=w650:refnum<queue>)  [unwired: 2 in, 2 out]
                }
              }
            }
          }
          frame 13 {
            # ">>> yStepper command>>>"
            # ">> Manual override >>"
            n252 = Dequeue Element(queue=w660, timeout in ms (-1)=w659, error in (no error)=w661) -> (element=w658:T7)  [unwired: 3 out]
            n253 = Equal?(x=w657, y=u8 80) -> (x = y?=w655:bool)
            n254 = case shown="\"None\", Default" w658 {
              tunnel: [w671 State_Type_Definitions."True Stop" ("Enum")] -> w662
              tunnel: [w674 w691] -> w663
              tunnel: [State_Type_Definitions."Idle" ("Enum") State_Type_Definitions."Shutdown" ("Enum")] -> w664
              tunnel: w655 -> [w670 _]
              tunnel: w654 -> [w669 _]
              tunnel: w653 -> [w665 w688]
              frame "None", Default {
                # "Stays in Task 5_A until stepper reaches desired \nheight"
                # "T: Go back to idle, F: Continue with task\""
                # ">> Manual override >>"
                n255 = case shown="True" w670 {
                  tunnel: [w678 w684] -> w674
                  tunnel: w665 -> [w676 w682]
                  frame False {
                    n256 = for {
                      tunnel: string[] ["Z STEPPER CAM HEIGHT", "READ STEPPER VALUES"] ("element") -> [w679] mode=indexing
                      shift-right: [w681] -> w678
                      shift-left: w676 -> [w680]
                      n257 = Enqueue Element(queue=w680, element=w679) -> (queue out=w681:refnum<queue>)  [unwired: 2 in, 2 out]
                    }
                  }
                  frame True {
                    n258 = for {
                      shift-right: [w686] -> w684
                      shift-left: w682 -> [w687]
                      tunnel: string[] ["OPEN LOG CAM", "SET TIMER", ""] -> [w685] mode=indexing
                      n259 = Enqueue Element(queue=w687, element=w685) -> (queue out=w686:refnum<queue>)  [unwired: 2 in, 2 out]
                    }
                  }
                }
                n260 = Or(x=w670, y=w669) -> (x .or. y?=w672:bool)
                n261 = Select(t=State_Type_Definitions."True Stop" ("Enum"), s=w669, f=State_Type_Definitions."Task 5 _B" ("Enum")) -> (s? t:f=w666:u16)
                n262 = Select(t=w666, s=w672, f=State_Type_Definitions."Task 5_A" ("Enum")) -> (s? t:f=w671:u16)
              }
              frame "Exit" {
                n263 = for {
                  shift-right: [w694] -> w691
                  shift-left: w688 -> [w695]
                  tunnel: string[] ["STOP", "RESET ENCODERS", "RESET YAW", "ARDUINO MODE 0"] -> [w693] mode=indexing
                  n264 = Enqueue Element(queue=w695, element=w693) -> (queue out=w694:refnum<queue>)  [unwired: 2 in, 2 out]
                }
              }
            }
          }
          frame 14 {
            # ">>> yStepper command>>>"
            n265 = Dequeue Element(queue=w699, timeout in ms (-1)=w698, error in (no error)=w700) -> (element=w697:T7)  [unwired: 3 out]
            n266 = And(x=w702, y=w703) -> (x .and. y?=w701:bool)
            "Recognized object + Time up?" <- w701
            n267 = case shown="\"None\", Default" w697 {
              tunnel: [w715 State_Type_Definitions."True Stop" ("Enum")] -> w705
              tunnel: [w718 w735] -> w704
              tunnel: [State_Type_Definitions."Idle" ("Enum") State_Type_Definitions."Shutdown" ("Enum")] -> w706
              tunnel: w701 -> [w714 _]
              tunnel: w708 -> [w713 _]
              tunnel: w707 -> [w709 w732]
              frame "None", Default {
                # "Stays in Task 5_B until time is up and object is detected"
                # "T: Go back to idle, F: Continue with task\""
                # ">> Manual override >>"
                n268 = case shown="True" w714 {
                  tunnel: [w722 w728] -> w718
                  tunnel: w709 -> [w720 w726]
                  frame False {
                    n269 = for {
                      tunnel: string[] ["CAM ACQ", "START TIMER"] ("element") -> [w723] mode=indexing
                      shift-right: [w725] -> w722
                      shift-left: w720 -> [w724]
                      n270 = Enqueue Element(queue=w724, element=w723) -> (queue out=w725:refnum<queue>)  [unwired: 2 in, 2 out]
                    }
                  }
                  frame True {
                    n271 = for {
                      shift-right: [w730] -> w728
                      shift-left: w726 -> [w731]
                      tunnel: string[] ["CAM CLOSE", ""] -> [w729] mode=indexing
                      n272 = Enqueue Element(queue=w731, element=w729) -> (queue out=w730:refnum<queue>)  [unwired: 2 in, 2 out]
                    }
                  }
                }
                n273 = Or(x=w714, y=w713) -> (x .or. y?=w716:bool)
                n274 = Select(t=State_Type_Definitions."True Stop" ("Enum"), s=w713, f=State_Type_Definitions."Task 5_C" ("Enum")) -> (s? t:f=w710:u16)
                n275 = Select(t=w710, s=w716, f=State_Type_Definitions."Task 5 _B" ("Enum")) -> (s? t:f=w715:u16)
              }
              frame "Exit" {
                n276 = for {
                  shift-right: [w738] -> w735
                  shift-left: w732 -> [w739]
                  tunnel: string[] ["STOP", "RESET ENCODERS", "RESET YAW", "ARDUINO MODE 0"] -> [w737] mode=indexing
                  n277 = Enqueue Element(queue=w739, element=w737) -> (queue out=w738:refnum<queue>)  [unwired: 2 in, 2 out]
                }
              }
            }
          }
          frame 15 {
            # ">>> yStepper command>>>"
            # ">> Checks if item is in range >>"
            # ">> Manual override >>"
            n278 = Dequeue Element(queue=w751, timeout in ms (-1)=w750, error in (no error)=w749) -> (element=w748:T7)  [unwired: 3 out]
            n279 = In Range and Coerce(upper limit=290.0, x=w744, lower limit=300.0) -> (In Range?=w741:bool)  [unwired: 1 out]
            n280 = case shown="\"None\", Default" w748 {
              tunnel: [w758 State_Type_Definitions."True Stop" ("Enum")] -> w753
              tunnel: [w761 w778] -> w746
              tunnel: [State_Type_Definitions."Idle" ("Enum") State_Type_Definitions."Shutdown" ("Enum")] -> w745
              tunnel: w741 -> [w757 _]
              tunnel: w747 -> [w756 _]
              tunnel: w752 -> [w755 w775]
              frame "None", Default {
                # ">> Is object in range? >>"
                # "Stays in Task 5_C until time is up and object is detected"
                # ">> Manual override >>"
                n281 = case shown="False" w757 {
                  tunnel: [w765 w771] -> w761
                  tunnel: w755 -> [w763 w769]
                  frame False {
                    n282 = for {
                      tunnel: string[] ["CAM ACQ", "START TIMER"] ("element") -> [w766] mode=indexing
                      shift-right: [w768] -> w765
                      shift-left: w763 -> [w767]
                      n283 = Enqueue Element(queue=w767, element=w766) -> (queue out=w768:refnum<queue>)  [unwired: 2 in, 2 out]
                    }
                  }
                  frame True {
                    n284 = for {
                      shift-right: [w773] -> w771
                      shift-left: w769 -> [w774]
                      tunnel: string[] ["CAM CLOSE", ""] -> [w772] mode=indexing
                      n285 = Enqueue Element(queue=w774, element=w772) -> (queue out=w773:refnum<queue>)  [unwired: 2 in, 2 out]
                    }
                  }
                }
                n286 = Or(x=w757, y=w756) -> (x .or. y?=w759:bool)
                n287 = Select(t=State_Type_Definitions."True Stop" ("Enum"), s=w759, f=State_Type_Definitions."Task 5_C_Error" ("Enum")) -> (s? t:f=w758:u16)
              }
              frame "Exit" {
                n288 = for {
                  shift-right: [w781] -> w778
                  shift-left: w775 -> [w782]
                  tunnel: string[] ["STOP", "RESET ENCODERS", "RESET YAW", "ARDUINO MODE 0"] -> [w780] mode=indexing
                  n289 = Enqueue Element(queue=w782, element=w780) -> (queue out=w781:refnum<queue>)  [unwired: 2 in, 2 out]
                }
              }
            }
          }
          frame 16 {
            # ">>> yStepper command>>>"
            # ">> Checks if yStepper has reached target>>"
            n290 = Dequeue Element(queue=w793, timeout in ms (-1)=w792, error in (no error)=w791) -> (element=w790:T7)  [unwired: 3 out]
            n291 = formula code="if (pos < 130)\ny = 30;\n\nelse if (pos >= 130 && pos <= 320)\ny = 15;\n\nelse if (pos > 320)\ny = 0;\n\nelse\ny  = 0;"("pos"=w783) -> ("y"=w787:dbl)
            n292 = To Unsigned Byte Integer(number=w787) -> (unsigned 8bit integer=w785:u8)
            n293 = Equal?(x=w786, y=w785) -> (x = y?=w784:bool)
            n294 = case shown="\"None\", Default" w790 {
              tunnel: [w805 State_Type_Definitions."True Stop" ("Enum")] -> w797
              tunnel: [w808 w825] -> w796
              tunnel: [State_Type_Definitions."Idle" ("Enum") State_Type_Definitions."Shutdown" ("Enum")] -> w798
              tunnel: w794 -> [w804 _]
              tunnel: w795 -> [w800 w822]
              tunnel: w784 -> [w799 _]
              frame "None", Default {
                # ">> T: Breaks out of state loop; F: Stays in loop>>"
                # ">> Manual override >>"
                # ">> Checks if yStepper has reached target>>"
                # "Stays in Task 5_C until time is up and object is detected"
                # "T: Go back to idle, F: Continue with task\""
                # ">> Manual override >>"
                n295 = case shown="True" w799 {
                  tunnel: [w812 w818] -> w808
                  tunnel: w800 -> [w810 w816]
                  frame False {
                    n296 = for {
                      tunnel: string[] ["Y STEPPER CONTROL", "READ STEPPER VALUES"] ("element") -> [w813] mode=indexing
                      shift-right: [w815] -> w812
                      shift-left: w810 -> [w814]
                      n297 = Enqueue Element(queue=w814, element=w813) -> (queue out=w815:refnum<queue>)  [unwired: 2 in, 2 out]
                    }
                  }
                  frame True {
                    n298 = for {
                      shift-right: [w820] -> w818
                      shift-left: w816 -> [w821]
                      tunnel: string[] ["OPEN LOG CAM", ""] -> [w819] mode=indexing
                      n299 = Enqueue Element(queue=w821, element=w819) -> (queue out=w820:refnum<queue>)  [unwired: 2 in, 2 out]
                    }
                  }
                }
                n300 = Or(x=w799, y=w804) -> (x .or. y?=w806:bool)
                n301 = Select(t=State_Type_Definitions."True Stop" ("Enum"), s=w804, f=State_Type_Definitions."Task 5 _B" ("Enum")) -> (s? t:f=w801:u16)
                n302 = Select(t=w801, s=w806, f=State_Type_Definitions."Task 5_C_Error" ("Enum")) -> (s? t:f=w805:u16)
              }
              frame "Exit" {
                n303 = for {
                  shift-right: [w828] -> w825
                  shift-left: w822 -> [w829]
                  tunnel: string[] ["STOP", "RESET ENCODERS", "RESET YAW", "ARDUINO MODE 0"] -> [w827] mode=indexing
                  n304 = Enqueue Element(queue=w829, element=w827) -> (queue out=w828:refnum<queue>)  [unwired: 2 in, 2 out]
                }
              }
            }
            n305 = Bundle By Name(cluster=w789, "yStepper desired"=w785) -> (w788:T8)
          }
          frame 23 {
            # ">>> yStepper command>>>"
            n306 = Dequeue Element(queue=w837, timeout in ms (-1)=w836, error in (no error)=w835) -> (element=w842:T7)  [unwired: 3 out]
            n307 = Equal?(x=w833, y=u8 80) -> (x = y?=w832:bool)
            n308 = case shown="\"None\", Default" w842 {
              tunnel: [w849 State_Type_Definitions."True Stop" ("Enum")] -> w840
              tunnel: [w848 w866] -> w839
              tunnel: [State_Type_Definitions."Idle" ("Enum") State_Type_Definitions."Shutdown" ("Enum")] -> w841
              tunnel: w838 -> [w844 _]
              tunnel: w834 -> [w846 _]
              tunnel: w832 -> [w843 _]
              frame "None", Default {
                n309 = case shown="False" w843 {
                  tunnel: [w854 w860] -> w848
                  tunnel: w846 -> [w852 w858]
                  frame False {
                    n310 = for {
                      tunnel: string[] ["Z STEPPER CAM HEIGHT", "READ STEPPER VALUES"] ("element") -> [w855] mode=indexing
                      shift-right: [w857] -> w854
                      shift-left: w852 -> [w856]
                      n311 = Enqueue Element(queue=w856, element=w855) -> (queue out=w857:refnum<queue>)  [unwired: 2 in, 2 out]
                    }
                  }
                  frame True {
                    n312 = for {
                      shift-right: [w862] -> w860
                      shift-left: w858 -> [w863]
                      tunnel: string[] ["CAM ACQ", ""] -> [w861] mode=indexing
                      n313 = Enqueue Element(queue=w863, element=w861) -> (queue out=w862:refnum<queue>)  [unwired: 2 in, 2 out]
                    }
                  }
                }
                n314 = Or(x=w843, y=w844) -> (x .or. y?=w845:bool)
                n315 = Select(t=State_Type_Definitions."Task 6_B" ("Enum"), s=w845, f=State_Type_Definitions."Task 6_A" ("Enum")) -> (s? t:f=w849:T6)
              }
              frame "Exit" {
                n316 = for {
                  shift-right: [w869] -> w866
                  shift-left: _ -> [w870]
                  tunnel: string[] ["STOP", "RESET ENCODERS", "RESET YAW", "ARDUINO MODE 0"] -> [w868] mode=indexing
                  n317 = Enqueue Element(queue=w870, element=w868) -> (queue out=w869:refnum<queue>)  [unwired: 2 in, 2 out]
                }
              }
            }
          }
          frame 24 {
            # ">>> yStepper command>>>"
            n318 = Dequeue Element(queue=w880, timeout in ms (-1)=w878, error in (no error)=w879) -> (element=w877:T7)  [unwired: 3 out]
            n319 = case shown="\"None\", Default" w877 {
              tunnel: [w887 State_Type_Definitions."True Stop" ("Enum")] -> w873
              tunnel: [w886 w905] -> w881
              tunnel: [State_Type_Definitions."Idle" ("Enum") State_Type_Definitions."Shutdown" ("Enum")] -> w874
              tunnel: w876 -> [w882 _]
              tunnel: w875 -> [w884 _]
              tunnel: w872 -> [w883 w902]
              frame "None", Default {
                # ">> Manual override >>"
                n320 = case shown="True" w884 {
                  tunnel: [w892 w898] -> w886
                  tunnel: w883 -> [w891 w896]
                  frame False {
                    n321 = for {
                      shift-right: [w895] -> w892
                      shift-left: w891 -> [w894]
                      tunnel: string[] ["CAM ACQ", "OPEN CLAW"] -> [w893] mode=indexing
                      n322 = Enqueue Element(queue=w894, element=w893) -> (queue out=w895:refnum<queue>)  [unwired: 2 in, 2 out]
                    }
                  }
                  frame True {
                    n323 = for {
                      shift-right: [w900] -> w898
                      shift-left: w896 -> [w901]
                      tunnel: string[] ["CAM ACQ", "CLOSE CLAW"] -> [w899] mode=indexing
                      n324 = Enqueue Element(queue=w901, element=w899) -> (queue out=w900:refnum<queue>)  [unwired: 2 in, 2 out]
                    }
                  }
                }
                n325 = Select(t=State_Type_Definitions."True Stop" ("Enum"), s=w882, f=State_Type_Definitions."Task 6_B" ("Enum")) -> (s? t:f=w887:T6)
              }
              frame "Exit" {
                # ">> State after true stop >>"
                # ">> Goes to true stop >>"
                n326 = for {
                  shift-right: [w908] -> w905
                  shift-left: w902 -> [w909]
                  tunnel: string[] ["STOP", "RESET ENCODERS", "RESET YAW", ""] -> [w907] mode=indexing
                  n327 = Enqueue Element(queue=w909, element=w907) -> (queue out=w908:refnum<queue>)  [unwired: 2 in, 2 out]
                }
              }
            }
          }
        }
      }
    }
  }
  n328 = call <vilib>:"DIO Close.vi"("error in (no error)"=w24, "DIO Info In"=w27) -> ()  [unwired: 9 in, 1 out]
  n329 = call <vilib>:"DIO Close.vi"("error in (no error)"=w34, "DIO Info In"=w36) -> ()  [unwired: 9 in, 1 out]
  n330 = call <vilib>:"NavX Close.vi"("error in (no error)"=w5, "NavX Info In"=w4) -> ()  [unwired: 9 in, 1 out]
  n331 = call <vilib>:"DIO Close.vi"("error in (no error)"=w29, "DIO Info In"=w31) -> ()  [unwired: 9 in, 1 out]
  n332 = call <vilib>:"DIO Close.vi"("error in (no error)"=w12, "DIO Info In"=w13) -> ()  [unwired: 9 in, 1 out]
  n333 = call <vilib>:"DIO Close.vi"("error in (no error)"=w7, "DIO Info In"=w8) -> ()  [unwired: 9 in, 1 out]
  n334 = while {
    stop <- w1323 stop-if-true
    n335 = call <vilib>:"RT Get CPU Loads.vi"() -> ("CPU loads"=→"CPU loads":T5[])  [unwired: 10 in, 1 out]
    n336 = Wait (ms)(milliseconds to wait=u32 100) -> ()  [unwired: 1 out]
    n337 = call "FGV Bool.vi"("Init/Read/Write State"=States_for_Action_Engine."Read") -> ("Output node"=w1323:bool)  [unwired: 2 in, 1 out]
  }
  n338 = Merge Errors "Merge Errors"(w64, w63) -> (w46:errorcluster)
  n339 = Merge Errors(w50, w46) -> (w45:errorcluster)
  n340 = Destroy User Event(user event=w67, error in=w45) -> ()  [unwired: 1 out]
  n341 = Destroy User Event(user event=w68, error in=w45) -> ()  [unwired: 1 out]
  n342 = Unregister For Events(event registration refnum=w59, error in=w45) -> ()  [unwired: 1 out]
  n343 = Release Queue(queue=w41, error in (no error)=w45) -> (error out=w23:errorcluster)  [unwired: 1 in, 2 out]
  n344 = Release Queue(queue=w58, error in (no error)=w45) -> ()  [unwired: 1 in, 3 out]
  n345 = call <vilib>:"Simple Error Handler.vi"("error in (no error)"=w23) -> ("error out"=w22:errorcluster)  [unwired: 4 in, 4 out]
  n346 = call <vilib>:"Reset myRIO.vi"("error in (no error)"=w22) -> ("error out"=→"error out":errorcluster)  [unwired: 10 in]
